vi "Execute_Analysis.vi"(0 "Image In":T2, 1 "ProjectName":string, 5 "Coordinate System Out (Set Coordinate System 1)":T3 {"Measurement System"."Axis Reference" items=["Direct", "Indirect"]; "Measurement System"."Angle (deg)" format="%.2f"; "Measurement System"."Origin"."Y" format="%.2f"; "Measurement System"."Origin"."X" format="%.2f"; "Reference System"."Axis Reference" items=["Direct", "Indirect"]; "Reference System"."Angle (deg)" format="%.2f"; "Reference System"."Origin"."Y" format="%.2f"; "Reference System"."Origin"."X" format="%.2f"}, 7 "ForCalCalculaton In":T2, 9 "ROI Entry":T4={"vROIName"="", "vROIContour"={"Contour Type"=0, "ROI Type"=0, "Points"=[]}, "ProcessSetting"=[], "Analysis_Setting"={"PreProcess"=enum."*Algorithm*", "Parameter"=""}}, 11 "error in (no error)":errorcluster, 12 "RootPath":path, 13 "CreatDllImage":bool, 14 "Script Index":i32) -> (4 "Image Out":T2, 6 "Result":variant, 8 "Analysis_Point_Result Out Overlay":T1[](array[typedef]), 10 "Analysis_Point_Result Out":T1[](array[typedef]), 15 "error out":errorcluster)   [LabVIEW 2019]
uses:
  Controls/Parttern Match/Analysis_PatternMatch_Parameter.ctl
  Controls/Barcode 1D/Analysis_Barcode 1D_Parameter.ctl
  <vilib>/vision/Instrument.llb/Demodulation Mode.ctl
  <vilib>/vision/Instrument.llb/Cell Sample Size.ctl
  <vilib>/vision/Instrument.llb/Cell Filter Mode.ctl
  <vilib>/vision/Instrument.llb/QR Code Search Options.ctl
  <vilib>/vision/Instrument.llb/Data Matrix Polarity.ctl
  <vilib>/vision/Instrument.llb/QR Code Model Type.ctl
  <vilib>/vision/Instrument.llb/QR Code Description Options.ctl
  Controls/Barcode 2D/Analysis_Barcode 2D_Parameter.ctl
  Controls/Clamp/Analysis_Clamp_Parameter.ctl
  Controls/Clamp MAX/Analysis_Clamp MAX_Parameter.ctl
  Controls/Particle/Analysis_Particle_Parameter.ctl
  Controls/Edge Detection/Analysis_Edge Detection_Parameter.ctl
  <vilib>/vision/NI_Vision_Development_Module.lvlib
  <vilib>/vision/Measure.llb/Edge Polarity.ctl
  <vilib>/vision/Measure.llb/Edge Options.ctl
  <vilib>/vision/Measure.llb/Straight Edge Process.ctl
  <vilib>/vision/Measure.llb/Straight Edge Options.ctl
  Controls/Find Straight Edge/Analysis_Find Straight Edge_Parameter.ctl
  <vilib>/vision/Instrument.llb/Data Matrix Search Options.ctl
  <vilib>/vision/Instrument.llb/Data Matrix Mirror.ctl
  <vilib>/vision/Instrument.llb/Cell Fill Percentage.ctl
  <vilib>/vision/Instrument.llb/ECC Type.ctl
  <vilib>/vision/Instrument.llb/Data Matrix Description Options.ctl
  DLL/[Global] Template.vi
  <vilib>/vision/Measure.llb/Edge New.ctl
  Controls/Parameter.ctl
  Controls/Histogram/Analysis_Histogram_Parameter.ctl
  Controls/Circle/Analysis_Circle_Parameter.ctl
  Controls/Parttern Match/Analysis_PatternMatch_ResultWithnumber.ctl
  Controls/ShapeDectect/Analysis_ShapeDectect_Parameter.ctl
  Controls/OCR/Analysis_OCR_Setting Parameter.ctl
  <vilib>/vision/Contour.llb/IMAQ Contour Curve Extraction.ctl
  <vilib>/vision/Contour.llb/IMAQ Connect Range Setting.ctl
  Controls/Contour/Analysis_Contour_Parameter.ctl
  Controls/ColorMatch/Analysis_ColorMatch_Parameter.ctl
  Controls/ColorMatch/Analysis_ColorMatch_Result.ctl
  <vilib>/vision/Instrument.llb/Data Matrix Advanced Options.ctl
  <vilib>/vision/Instrument.llb/Data Matrix Size Options.ctl
  Controls/Analysis_Type.ctl
  <vilib>/vision/Image Controls.llb/IMAQ Image.ctl
  Controls/Analysis_Setting.ctl
  Process/Controls/Process_Setting.ctl
  Controls/Vision_DataEntry.ctl
  Controls/Analysis_Result_To_Caliper.ctl
  Ctrl/VisionProcessName.ctl
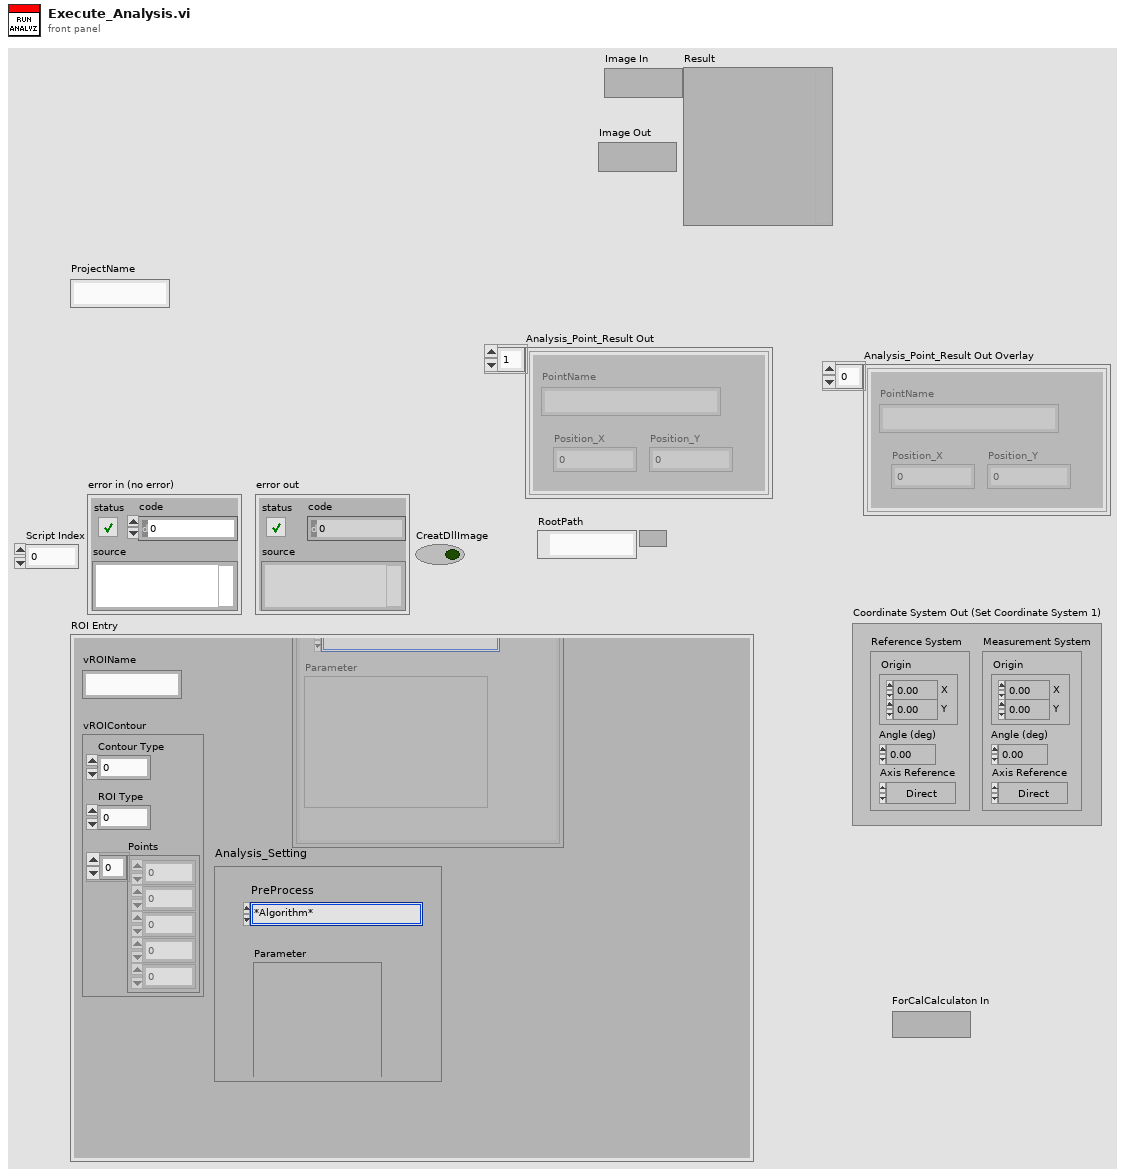
[diagram p1: front panel]
types:
  T1 = typedef "Analysis_Result_To_Caliper.ctl" = cluster{"PointName":string, "Position_X":dbl, "Position_Y":dbl}
  T2 = typedef "IMAQ Image.ctl" = refnum<image>
  T3 = cluster{"Reference System":cluster{"Origin":cluster{"X":sgl, "Y":sgl}, "Angle (deg)":sgl, "Axis Reference":u32}, "Measurement System":cluster{"Origin":cluster{"X":sgl, "Y":sgl}, "Angle (deg)":sgl, "Axis Reference":u32}}
  T4 = typedef "Vision_DataEntry.ctl" = cluster{"vROIName":string, "vROIContour":cluster{"Contour Type":u32, "ROI Type":u32, "Points":i32[]}, "ProcessSetting":T5[], "Analysis_Setting":T7}
  T5 = typedef "Process_Setting.ctl" = cluster{"Enum_PreProcess":T6, "Parameter":string}
  T6 = typedef "VisionProcessName.ctl" = enum16{"*CamParameter*", "CamAttributes", "*Preprocess*", "CG_Brightness", "C_Plane Extraction", "C_Threshold", "G_Lookup Table", "G_Threshold"}
  T7 = typedef "Analysis_Setting.ctl" = cluster{"PreProcess":T8, "Parameter":string}
  T8 = typedef "VisionProcessName.ctl" = enum16{"*CamParameter*", "CamAttributes", "*Preprocess*", "CG_Brightness", "C_Plane Extraction", "C_Threshold", "G_Lookup Table", "G_Threshold", "B_Image Inversion", "*Algorithm*", "CG_Histogram", "C_Color Matching", "C_Color Pattern Matching", "G_PatternMatch", "CG_Find Straight Edge", "CG_Adv. Find Straight Edge", "CG_Find Circular Edge", "G_Max Clamp", "G_Clamp (Rake)", "G_Pattern Matching"}
  T9 = typedef "Analysis_Type.ctl" = u16
  T10 = typedef "Parameter.ctl" = enum16{"Initialize", "Write", "Read", "WriteAll", "Save", "Load"}
  T11 = typedef "ParameterData.ctl" = cluster{"Rotate Angle":dbl, "Rotate?":bool, "Calibration File Path":string, "Cal?":bool}
  T12 = typedef "ROI Descriptor" = cluster{"Global Rectangle":i32[], "Contours":cluster{"ID":enum32{"External", "Internal"}, "Type":u32, "Coordinates":i32[]}[]}
  T13 = cluster{"Algorithm":i32, "Match Parameters":cluster{"Number of Matches Requested":i32, "Minimum Match Score":sgl, "Angle Ranges":cluster{"Start Angle":sgl, "End Angle":sgl}[]}, "ROI Descriptor":T12, "Advanced Options":cluster{"Item":u16, "Value":dbl}[], "Template path":string}
  T14 = typedef "Analysis_PatternMatch_ResultWithnumber.ctl" = cluster{"numbers":i32, "results":cluster{"ROI Descriptor out":T12, "Point":T15, "Angle":sgl, "Score":sgl, "Real World Coordinates":cluster{"X":sgl, "Y":sgl}, "Rectangle":T16}[]}
  T15 = typedef "IMAQ Point" = cluster{"X":sgl, "Y":sgl}
  T16 = typedef "IMAQ Rectangle" = cluster{"Left":i32, "Top":i32, "Right":i32, "Bottom":i32, "Rotation":dbl}
  T17 = typedef "Edge New.ctl" = cluster{"Location (Pixel)":cluster{"X":sgl, "Y":sgl}, "Location (Real-World)":cluster{"X":sgl, "Y":sgl}, "Distance (Pixel)":dbl, "Distance (Real-World)":dbl, "Strength":dbl, "Noise":dbl, "Rising?":bool}
  T18 = cluster{"Edge Information":T17[], "Number of Edges Detected":i32}
  T19 = cluster{cluster{"x":sgl, "y":sgl}[][], string[], "Barcodes":cluster{"Data":string, "Special Char 1":string, "Special Char 2":string, "Checksum(s)":string, "Barcode Type":u32, "Confidence Level":sgl, "Bounding Box":cluster{"x":sgl, "y":sgl}[]}[]}
  T20 = cluster{"Data":string, cluster{"x":sgl, "y":sgl}[]}
  T21 = cluster{"Points":cluster{"X":sgl, "Y":sgl}[], "Perpendicular Lines":cluster{cluster{sgl, sgl}, cluster{sgl, sgl}}[], "appended array":cluster{"X":sgl, "Y":sgl}[], "Line Coordinates":cluster{cluster{sgl, sgl}, cluster{sgl, sgl}}[], "Clamp Settings":cluster{"Contrast":i32, "Filter width":i32, "Steepness":i32, "Subsampling Ratio":u32, "Show Search Area":bool, "Show Search Lines":bool, "Show Edges Found":bool, "Show Result":bool}, "ROI Descriptor":cluster{"Global Rectangle":i32[], "Contours":cluster{"Contour Type":u32, "ROI Type":u32, "Points":i32[]}[]}, "Distance":sgl, "Edge Coordinates":cluster{"X":sgl, "Y":sgl}[], "Edge Coordinates  (Real World)":cluster{"X":sgl, "Y":sgl}[], "Distance (Real World)":sgl}
  T22 = cluster{cluster{"X":sgl, "Y":sgl}, cluster{"X":sgl, "Y":sgl}}
  T23 = cluster{"Area":dbl, "Number of Holes":dbl, "Bounding Rect":cluster{"Left":dbl, "Top":dbl, "Right":dbl, "Bottom":dbl}, "Center of Mass":cluster{"X":dbl, "Y":dbl}, "Orientation":dbl, "Dimensions":cluster{"Width":dbl, "Height":dbl}}
  T24 = cluster{"Left":dbl, "Top":dbl, "Right":dbl, "Bottom":dbl}
  T25 = cluster{"Point1 (Pixels)":cluster{"X":sgl, "Y":sgl}, "Point2 (Pixels)":cluster{"X":sgl, "Y":sgl}, "Point1 (Real-World)":cluster{"X":sgl, "Y":sgl}, "Point2 (Real-World)":cluster{"X":sgl, "Y":sgl}, "Angle (Pixel)":dbl, "Angle (Real-World)":dbl, "Score":dbl, "Straightness":dbl, "Average SNR (db)":dbl, "Calibration Valid":bool}
  T26 = typedef "IMAQ Circle" = cluster{"Center X":i32, "Center Y":i32, "Inner Radius":i32, "Outer Radius":i32, "Start Angle":dbl, "End Angle":dbl}
  T27 = typedef "Analysis_ShapeDectect_Parameter.ctl" = cluster{"Enum_ShapeType":enum16{"Circles", "Ellipses", "Lines", "Rectangles"}, "MaxParticle":i32, "Descriptor":cluster{"Set 1":dbl, "Set 2":dbl, "Set 3":dbl, "Set 4":dbl}, "Match Options":cluster{"Rotation":bool, "Scale":bool, "Occlusion":bool, "Range Settings":cluster{"Match Constraints":u32, "Min":dbl, "Max":dbl}[]}, "Curve Parameters":cluster{"Extraction Mode":u32, "Edge Threshold":i32, "Edge Filter Size":u32, "Min Length":i32, "Row Search Step Size":i32, "Col Search Step Size":i32, "Max Endpoint Gap":i32, "Closed":bool, "Subpixel":bool}, " score":dbl}
  T28 = typedef "Analysis_OCR_Setting Parameter.ctl" = cluster{"OCRSelectedLanaguage":string[]}
  T29 = typedef "Analysis_ColorMatch_Result.ctl" = cluster{"Match Flag":bool[], "Match Score":i32[], "ROI Descriptor":T12}
  T30 = typedef "Analysis_ColorMatch_Parameter.ctl" = cluster{"Color Sensitivity":u32, "Learn Saturation Threshold":i32, "Minimum Match Score":dbl, "Match Saturation Threshold":i32, "ROI Descriptor":T12, "TemplatePath":string, "ColorSpectrum":dbl[]}
  T31 = typedef "Analysis_PatternMatch_Parameter.ctl" = cluster{"Algorithm":i32, "Match Parameters":cluster{"Number of Matches Requested":i32, "Minimum Match Score":sgl, "Angle Ranges":cluster{"Start Angle":sgl, "End Angle":sgl}[]}, "ROI Descriptor":T12, "Advanced Options":cluster{"Item":u16, "Value":dbl}[], "Template path":string, "XOffset":i32, "YOffset":i32}
  T32 = typedef "Image Type" = u32
  T33 = cluster{"Number of Matches Requested":i32, "Minimum Match Score":sgl, "Angle Ranges":cluster{"Start Angle":sgl, "End Angle":sgl}[]}
  T34 = cluster{"Script Name":string, "TemplateArray":cluster{"ROI Name":string, "TemplateImage":T2}[]}[]
  T35 = cluster{"Script Name":string, "TemplateArray":cluster{"ROI Name":string, "TemplateImage":T2}[]}
  T36 = cluster{"Origin":cluster{"X":sgl, "Y":sgl}, "Angle (deg)":sgl, "Axis Reference":u32}
  T37 = typedef "Analysis_PatternMatch_Result.ctl" = cluster{"Position":cluster{"x":sgl, "y":sgl}, "Angle":sgl, "Scale":sgl, "Score":sgl, "Bounding Box":cluster{"x":sgl, "y":sgl}[]}
  T38 = cluster{"ROI Descriptor out":T12, "Point":T15, "Angle":sgl, "Score":sgl, "Real World Coordinates":cluster{"X":sgl, "Y":sgl}, "Rectangle":T16}
  T39 = typedef "Analysis_Edge Detection_Parameter.ctl" = cluster{"Edge Options":cluster{"Edge Polarity":u16, "Kernel Size":u32, "Width":u32, "Minimum Edge Strength":dbl, "Interpolation Type":u16, "Data Processing Method":u16}, "Process":u16, "Number of Matches Requested":i32, "ROI Descriptor":cluster{"Global Rectangle":i32[], "Contours":cluster{"Contour Type":u32, "ROI Type":u32, "Points":i32[]}[]}}
  T40 = cluster{"Edge Polarity":u16, "Kernel Size":u32, "Width":u32, "Minimum Edge Strength":dbl, "Interpolation Type":u16, "Data Processing Method":u16}
  T41 = cluster{"Global Rectangle":i32[], "Contours":cluster{"Contour Type":u32, "ROI Type":u32, "Points":i32[]}[]}
  T42 = cluster{"Contour Type":u32, "ROI Type":u32, "Points":i32[]}[]
  T43 = cluster{"Contour Type":u32, "ROI Type":u32, "Points":i32[]}
  T44 = typedef "Analysis_Barcode 1D_Parameter.ctl" = cluster{"Barcode Search Options":cluster{"Min Bar Width":dbl, "Min Edge Strength":dbl, "Min Bars":dbl, "Skip Location Search?":bool}, "Barcode Types To Search":enum16{"Reserved", "Codabar", "Code 39", "Code 93", "Code 128", "EAN 8", "EAN 13", "Interleaved 2 of 5", "MSI", "UPCA", "Pharmacode", "RSS Limited"}[], "Barcode Grading Options":cluster{"Calculate Grading Report":bool, "Scan Width ":dbl}, "Number of Matches Requested":i32, "ROI":cluster{"Global Rectangle":i32[], "Contours":cluster{"Contour Type":u32, "ROI Type":u32, "Points":i32[]}[]}}
  T45 = cluster{"Min Bar Width":dbl, "Min Edge Strength":dbl, "Min Bars":dbl, "Skip Location Search?":bool}
  T46 = enum16{"Reserved", "Codabar", "Code 39", "Code 93", "Code 128", "EAN 8", "EAN 13", "Interleaved 2 of 5", "MSI", "UPCA", "Pharmacode", "RSS Limited"}[]
  T47 = cluster{"Calculate Grading Report":bool, "Scan Width ":dbl}
  T48 = cluster{"Data":string, "Special Char 1":string, "Special Char 2":string, "Checksum(s)":string, "Barcode Type":u32, "Confidence Level":sgl, "Bounding Box":cluster{"x":sgl, "y":sgl}[]}[]
  T49 = cluster{T15[][], string[], "Barcodes":cluster{"Data":string, "Special Char 1":string, "Special Char 2":string, "Checksum(s)":string, "Barcode Type":u32, "Confidence Level":sgl, "Bounding Box":cluster{"x":sgl, "y":sgl}[]}[]}
  T50 = typedef "Analysis_Barcode 2D_Parameter.ctl" = cluster{"ROI":cluster{"Global Rectangle":i32[], "Contours":cluster{"Contour Type":u32, "ROI Type":u32, "Points":i32[]}[]}, "Barcode Type":enum16{"Data Matrix", "PDF417", "QR Code"}, "Data Matrix Parameter":cluster{"Data Matrix Description Options":T51, "Data Matrix Search Options":T56, "Data Matrix Size Options":T60, "Advanced Options":T61[]}, "PDF147 Search Mode":T62, "QR Code Parameter":cluster{"QR Search Options":T63, "QR Description Options":T64, "QR Code Cell Size (pixels)":cluster{"Minimum Size":u32, "Maximum Size":u32}}}
  T51 = typedef "Data Matrix Description Options.ctl" = cluster{"Aspect Ratio":sgl, "Rows":u32, "Columns":u32, "Rectangle":bool, "ECC":T52, "Barcode Polarity":T53, "Cell Fill Percentage":T54, "Minimum Border Integrity %":sgl, "Mirror Mode":T55}
  T52 = typedef "ECC Type.ctl" = i32
  T53 = typedef "Data Matrix Polarity.ctl" = i32
  T54 = typedef "Cell Fill Percentage.ctl" = i32
  T55 = typedef "Data Matrix Mirror.ctl" = i32
  T56 = typedef "Data Matrix Search Options.ctl" = cluster{"Rotation Mode":enum32{"Unlimited", "0 Degrees", "90 Degrees", "180 Degrees", "270 Degrees"}, "Skip Location?":bool, "Edge Threshold":u32, "Demodulation Mode":T57, "Cell Sample Size":T58, "Cell Filter Mode":T59, "Skew Degrees Allowed":u32, "Maximum Iterations":u32, "Initial Search Vector Width":u32}
  T57 = typedef "Demodulation Mode.ctl" = i32
  T58 = typedef "Cell Sample Size.ctl" = i32
  T59 = typedef "Cell Filter Mode.ctl" = i32
  T60 = typedef "Data Matrix Size Options.ctl" = cluster{"Data Matrix Size":cluster{"Minimum Size":u32, "Maximum Size":u32}, "Quiet Zone Width":u32}
  T61 = typedef "Data Matrix Advanced Options.ctl" = cluster{"Option":enum32{"Line Detection", "HighLight Filter", "Aggressive", "FNC1", "Refine Bounding Box"}, " Value":dbl}
  T62 = typedef "PDF417 Search Mode" = enum32{"Multiple Barcodes", "Single Barcode, Conservative"}
  T63 = typedef "QR Code Search Options.ctl" = cluster{"Rotation Mode":enum32{"Unlimited", "0 Degrees", "90 Degrees", "180 Degrees", "270 Degrees"}, "Skip Location?":bool, "Edge Threshold":u32, "Demodulation Mode":T57, "Cell Sample Size":T58, "Cell Filter Mode":T59, "Skew Degrees Allowed":u32}
  T64 = typedef "QR Code Description Options.ctl" = cluster{"Matrix Size (cells)":i32, "Barcode Polarity":T53, "Mirror Mode":i32, "QR Model":T65}
  T65 = typedef "QR Code Model Type.ctl" = i32
  T66 = cluster{"Data":string, "Bounding Box":cluster{"x":sgl, "y":sgl}[]}
  T67 = typedef "Analysis_Clamp_Parameter.ctl" = cluster{"Clamp Settings":cluster{"Contrast":i32, "Filter width":i32, "Steepness":i32, "Subsampling Ratio":u32, "Show Search Area":bool, "Show Search Lines":bool, "Show Edges Found":bool, "Show Result":bool}, "ROI Descriptor":cluster{"Global Rectangle":i32[], "Contours":cluster{"Contour Type":u32, "ROI Type":u32, "Points":i32[]}[]}, "Process":u16}
  T68 = cluster{"Contrast":i32, "Filter width":i32, "Steepness":i32, "Subsampling Ratio":u32, "Show Search Area":bool, "Show Search Lines":bool, "Show Edges Found":bool, "Show Result":bool}
  T69 = cluster{cluster{"X":sgl, "Y":sgl}, cluster{"X":sgl, "Y":sgl}}[]
  T70 = typedef "Analysis_Clamp MAX_Parameter.ctl" = cluster{"Overlay Settings":cluster{"Show Search Area":bool, "Show Curves":bool, "Show Clamp Locations":bool, "Show Result":bool, "Search Area Color":u32, "Curves Color":u32, "Clamp Locations Color":u32, "Result Color":u32, "Overlay Group Name":string}, "Curve Extraction Settings":cluster{"Extraction Mode":u32, "Edge Threshold":i32, "Edge Filter Size":u32, "Min Length":i32, "Row Search Step Size":i32, "Col Search Step Size":i32, "Max Endpoint Gap":i32, "Closed":bool, "Subpixel":bool}, "Clamp Settings":cluster{"Angle Range (+/-)":dbl, "Edge Polarity":cluster{"Start":u32, "End":u32}}, "ROI":cluster{"Global Rectangle":i32[], "Contours":cluster{"Contour Type":u32, "ROI Type":u32, "Points":i32[]}[]}}
  T71 = cluster{"Show Search Area":bool, "Show Curves":bool, "Show Clamp Locations":bool, "Show Result":bool, "Search Area Color":u32, "Curves Color":u32, "Clamp Locations Color":u32, "Result Color":u32, "Overlay Group Name":string}
  T72 = cluster{"Extraction Mode":u32, "Edge Threshold":i32, "Edge Filter Size":u32, "Min Length":i32, "Row Search Step Size":i32, "Col Search Step Size":i32, "Max Endpoint Gap":i32, "Closed":bool, "Subpixel":bool}
  T73 = cluster{"Angle Range (+/-)":dbl, "Edge Polarity":cluster{"Start":u32, "End":u32}}
  T74 = cluster{"Pixels ":cluster{"Start":cluster{"X":dbl, "Y":dbl}, "End":cluster{"X":dbl, "Y":dbl}}, "Real World":cluster{"Start":cluster{"X":dbl, "Y":dbl}, "End":cluster{"X":dbl, "Y":dbl}}}
  T75 = cluster{"Distance (Pixels)":dbl, "Distance (Real World)":dbl, "Angle (Absolute)":dbl, "Angle (Relative)":dbl}
  T76 = cluster{"Clamp Results":cluster{"Distance (Pixels)":dbl, "Distance (Real World)":dbl, "Angle (Absolute)":dbl, "Angle (Relative)":dbl}, "Clamp Points":cluster{"Pixels ":cluster{"Start":cluster{"X":dbl, "Y":dbl}, "End":cluster{"X":dbl, "Y":dbl}}, "Real World":cluster{"Start":cluster{"X":dbl, "Y":dbl}, "End":cluster{"X":dbl, "Y":dbl}}}}
  T77 = cluster{"Start":cluster{"X":dbl, "Y":dbl}, "End":cluster{"X":dbl, "Y":dbl}}
  T78 = typedef "Analysis_Particle_Parameter.ctl" = cluster{"Selected Particle":i32, "Connectivity 4/8 (8)":bool, "MaxParticle":i32}
  T79 = cluster{"Area":dbl, "Number of Holes":dbl, "Bounding Rect":cluster{"Left":dbl, "Top":dbl, "Right":dbl, "Bottom":dbl}, "Center of Mass":cluster{"X":dbl, "Y":dbl}, "Orientation":dbl, "Dimensions":cluster{"Width":dbl, "Height":dbl}}[]
  T80 = cluster{cluster{"Area":dbl, "Number of Holes":dbl, "Bounding Rect":cluster{"Left":dbl, "Top":dbl, "Right":dbl, "Bottom":dbl}, "Center of Mass":cluster{"X":dbl, "Y":dbl}, "Orientation":dbl, "Dimensions":cluster{"Width":dbl, "Height":dbl}}[], cluster{"Area":dbl, "Number of Holes":dbl, "Bounding Rect":cluster{"Left":dbl, "Top":dbl, "Right":dbl, "Bottom":dbl}, "Center of Mass":cluster{"X":dbl, "Y":dbl}, "Orientation":dbl, "Dimensions":cluster{"Width":dbl, "Height":dbl}}[]}
  T81 = typedef "Analysis_Histogram_Parameter.ctl" = cluster{"Interval Range":cluster{"Minimum":sgl, "Maximum":sgl}, "ROI Out":cluster{"Global Rectangle":i32[], "Contours":cluster{"Contour Type":u32, "ROI Type":u32, "Points":i32[]}[]}, "Number of Classes":i32}
  T82 = cluster{"histogram":u32[], "Minimal Value":sgl, "Maximal Value":sgl, "Starting Value":sgl, "Interval Width":sgl, "Mean Value":sgl, "Standard  Variation":sgl, "Area (pixels)":i32}
  T83 = cluster{"Histogram Report":cluster{"histogram":u32[], "Minimal Value":sgl, "Maximal Value":sgl, "Starting Value":sgl, "Interval Width":sgl, "Mean Value":sgl, "Standard  Variation":sgl, "Area (pixels)":i32}, "ROI Out":cluster{"Global Rectangle":i32[], "Contours":cluster{"Contour Type":u32, "ROI Type":u32, "Points":i32[]}[]}}
  T84 = typedef "Analysis_Find Straight Edge_Parameter.ctl" = cluster{"ROI Descriptor":cluster{"Global Rectangle":i32[], "Contours":cluster{"Contour Type":u32, "ROI Type":u32, "Points":i32[]}[]}, "Number of Matches Requested":i32, "Edge Info Size":i32, "Options":cluster{"Search Direction":u32, "Edge Options":T85, "Show Search Area":bool, "Show Search Lines":bool, "Show Edges Found":bool, "Show Result":bool, "Search Area Color":u32, "Search Lines Color":u32, "Edge Locations Color":u32, "Result Color":u32, "Overlay Group Name":string}, "Line Fit Options":T87}
  T85 = typedef "Edge Options.ctl" = cluster{"Edge Polarity":T86, "Kernel Size":u32, "Width":u32, "Minimum Edge Strength":sgl, "Interpolation Type":enum32{"Zero Order", "Bilinear", "Quadratic", "Cubic", "Bilinear Fixed"}, "Data Processing Method":enum32{"Average", "Median"}}
  T86 = typedef "Edge Polarity.ctl" = u32
  T87 = typedef "Straight Edge Options.ctl" = cluster{"Number of Lines":i32, "Type":T88, "Min. Score":dbl, "Max. Score":dbl, "Orientation":dbl, "Angle Range":dbl, "Angle Tolerance":dbl, "Step Size":u32, "Min. SNR (db)":dbl, "Min. Points (%)":dbl, "Hough Iterations":i32}
  T88 = typedef "Straight Edge Process.ctl" = enum32{"First Edge Rake", "Best Edge Rake", "Hough Edge Rake", "First Edge Projection", "Best Edge Projection"}
  T89 = cluster{"Search Direction":u32, "Edge Options":T85, "Show Search Area":bool, "Show Search Lines":bool, "Show Edges Found":bool, "Show Result":bool, "Search Area Color":u32, "Search Lines Color":u32, "Edge Locations Color":u32, "Result Color":u32, "Overlay Group Name":string}
  T90 = cluster{"Point1 (Pixels)":cluster{"X":sgl, "Y":sgl}, "Point2 (Pixels)":cluster{"X":sgl, "Y":sgl}, "Point1 (Real-World)":cluster{"X":sgl, "Y":sgl}, "Point2 (Real-World)":cluster{"X":sgl, "Y":sgl}, "Angle (Pixel)":dbl, "Angle (Real-World)":dbl, "Score":dbl, "Straightness":dbl, "Average SNR (db)":dbl, "Calibration Valid":bool}[]
  T91 = typedef "Analysis_Circle_Parameter.ctl" = cluster{"ROI Descriptor":cluster{"Global Rectangle":i32[], "Contours":cluster{"Contour Type":u32, "ROI Type":u32, "Points":i32[]}[]}, "Options":cluster{"Search  Direction":u32, "Edge Options":T85, "Show Search Area":bool, "Show Search Lines":bool, "Show Edges Found":bool, "Show Result":bool, "Search Area Color":u32, "Search Lines Color":u32, "Edge Locations Color":u32, "Result Color":u32, "Overlay Group Name":string}, "Circle Fit Options":cluster{"Process":enum16{"Get First Edge", "Get First + Last Edge", "Get All Edges", "Get Best Edge"}, "Step Size":dbl, "Max Pixel Radius":i32}}
  T92 = cluster{"Search  Direction":u32, "Edge Options":T85, "Show Search Area":bool, "Show Search Lines":bool, "Show Edges Found":bool, "Show Result":bool, "Search Area Color":u32, "Search Lines Color":u32, "Edge Locations Color":u32, "Result Color":u32, "Overlay Group Name":string}
  T93 = cluster{"Process":enum16{"Get First Edge", "Get First + Last Edge", "Get All Edges", "Get Best Edge"}, "Step Size":dbl, "Max Pixel Radius":i32}
  T94 = cluster{"Center (Pixels)":cluster{"X":sgl, "Y":sgl}, "Radius (Pixels)":dbl, "Center (Real-World)":cluster{"X":sgl, "Y":sgl}, "Radius (Real-World)":dbl, "Roundness (Real-World)":dbl, "Average Strength":dbl, "Average SNR (dB)":dbl}
  T95 = cluster{"ROI Descriptor out":T12, "ROI Descriptor out":T12, "Fitted Circle":cluster{"Center (Pixels)":cluster{"X":sgl, "Y":sgl}, "Radius (Pixels)":dbl, "Center (Real-World)":cluster{"X":sgl, "Y":sgl}, "Radius (Real-World)":dbl, "Roundness (Real-World)":dbl, "Average Strength":dbl, "Average SNR (dB)":dbl}}
  T96 = cluster{"Pixel":cluster{"Position":cluster{"X":sgl, "Y":sgl}, "Angle":dbl, "Major Radius":dbl, "Minor Radius":dbl, "Score":dbl}[], "Ellipses (Calibrated)":cluster{"Position":cluster{"X":sgl, "Y":sgl}, "Orientation":dbl, "Major Radius":dbl, "Minor Radius":dbl, "Score":dbl}[]}
  T97 = enum16{"Circles", "Ellipses", "Lines", "Rectangles"}
  T98 = cluster{"Circles":cluster{"Position":cluster{"X":sgl, "Y":sgl}, "Radius":dbl, "Score":dbl}[], "Circles (Calibrated)":cluster{"Position":cluster{"X":sgl, "Y":sgl}, "Radius":dbl, "Score":dbl}[]}
  T99 = cluster{"Position":cluster{"X":sgl, "Y":sgl}, "Radius":dbl, "Score":dbl}[]
  T100 = cluster{"Position":cluster{"X":sgl, "Y":sgl}, "Radius":dbl, "Score":dbl}
  T101 = cluster{"ROI Descriptor out":T12, "Circle Descriptor":cluster{"Position":cluster{"X":sgl, "Y":sgl}, "Radius":dbl, "Score":dbl}, "Circle Descriptor":cluster{"Position":cluster{"X":sgl, "Y":sgl}, "Radius":dbl, "Score":dbl}}
  T102 = cluster{"Enum_ShapeType":enum16{"Circles", "Ellipses", "Lines", "Rectangles"}, "DectectItem":i32, cluster{"ROI Descriptor out":T12, "Circle Descriptor":cluster{"Position":cluster{"X":sgl, "Y":sgl}, "Radius":dbl, "Score":dbl}, "Circle Descriptor":cluster{"Position":cluster{"X":sgl, "Y":sgl}, "Radius":dbl, "Score":dbl}}[]}
  T103 = cluster{"Position":cluster{"X":sgl, "Y":sgl}, "Angle":dbl, "Major Radius":dbl, "Minor Radius":dbl, "Score":dbl}[]
  T104 = cluster{"Position":cluster{"X":sgl, "Y":sgl}, "Orientation":dbl, "Major Radius":dbl, "Minor Radius":dbl, "Score":dbl}[]
  T105 = cluster{"Position":cluster{"X":sgl, "Y":sgl}, "Angle":dbl, "Major Radius":dbl, "Minor Radius":dbl, "Score":dbl}
  T106 = cluster{"Position":cluster{"X":sgl, "Y":sgl}, "Orientation":dbl, "Major Radius":dbl, "Minor Radius":dbl, "Score":dbl}
  T107 = cluster{"ROI Descriptor out":T12, "Circle Descriptor":cluster{"Position":cluster{"X":sgl, "Y":sgl}, "Angle":dbl, "Major Radius":dbl, "Minor Radius":dbl, "Score":dbl}, "Circle Descriptor":cluster{"Position":cluster{"X":sgl, "Y":sgl}, "Orientation":dbl, "Major Radius":dbl, "Minor Radius":dbl, "Score":dbl}}
  T108 = cluster{"Enum_ShapeType":enum16{"Circles", "Ellipses", "Lines", "Rectangles"}, "DectectItem":i32, cluster{"ROI Descriptor out":T12, "Circle Descriptor":cluster{"Position":cluster{"X":sgl, "Y":sgl}, "Angle":dbl, "Major Radius":dbl, "Minor Radius":dbl, "Score":dbl}, "Circle Descriptor":cluster{"Position":cluster{"X":sgl, "Y":sgl}, "Orientation":dbl, "Major Radius":dbl, "Minor Radius":dbl, "Score":dbl}}[]}
  T109 = cluster{"Lines":cluster{"Start Point":cluster{"X":sgl, "Y":sgl}, "End Point":cluster{"X":sgl, "Y":sgl}, "Length":dbl, "Angle":dbl, "Score":dbl}[], "Lines Calibrated":cluster{"Start Point":cluster{"X":sgl, "Y":sgl}, "End Point":cluster{"X":sgl, "Y":sgl}, "Length":dbl, "Orientation":dbl, "Score":dbl}[]}
  T110 = cluster{"Start Point":cluster{"X":sgl, "Y":sgl}, "End Point":cluster{"X":sgl, "Y":sgl}, "Length":dbl, "Angle":dbl, "Score":dbl}[]
  T111 = cluster{"Start Point":cluster{"X":sgl, "Y":sgl}, "End Point":cluster{"X":sgl, "Y":sgl}, "Length":dbl, "Orientation":dbl, "Score":dbl}[]
  T112 = cluster{"Start Point":cluster{"X":sgl, "Y":sgl}, "End Point":cluster{"X":sgl, "Y":sgl}, "Length":dbl, "Angle":dbl, "Score":dbl}
  T113 = cluster{"Start Point":cluster{"X":sgl, "Y":sgl}, "End Point":cluster{"X":sgl, "Y":sgl}, "Length":dbl, "Orientation":dbl, "Score":dbl}
  T114 = cluster{"Circle Descriptor":cluster{"Start Point":cluster{"X":sgl, "Y":sgl}, "End Point":cluster{"X":sgl, "Y":sgl}, "Length":dbl, "Angle":dbl, "Score":dbl}, "Circle Descriptor":cluster{"Start Point":cluster{"X":sgl, "Y":sgl}, "End Point":cluster{"X":sgl, "Y":sgl}, "Length":dbl, "Orientation":dbl, "Score":dbl}}
  T115 = cluster{"Enum_ShapeType":enum16{"Circles", "Ellipses", "Lines", "Rectangles"}, "DectectItem":i32, cluster{"Circle Descriptor":cluster{"Start Point":cluster{"X":sgl, "Y":sgl}, "End Point":cluster{"X":sgl, "Y":sgl}, "Length":dbl, "Angle":dbl, "Score":dbl}, "Circle Descriptor":cluster{"Start Point":cluster{"X":sgl, "Y":sgl}, "End Point":cluster{"X":sgl, "Y":sgl}, "Length":dbl, "Orientation":dbl, "Score":dbl}}[]}
  T116 = cluster{"Rectangles":cluster{"Corners":cluster{"X":sgl, "Y":sgl}[], "Angle":dbl, "Width":dbl, "Height":dbl, "Score":dbl}[], "Rectangles Calibrated":cluster{"Corners":cluster{"X":sgl, "Y":sgl}[], "Angle":dbl, "Width":dbl, "Height":dbl, "Score":dbl}[]}
  T117 = cluster{"Corners":cluster{"X":sgl, "Y":sgl}[], "Angle":dbl, "Width":dbl, "Height":dbl, "Score":dbl}[]
  T118 = cluster{"Corners":cluster{"X":sgl, "Y":sgl}[], "Angle":dbl, "Width":dbl, "Height":dbl, "Score":dbl}
  T119 = cluster{"Rectangle Descriptor":cluster{"Corners":cluster{"X":sgl, "Y":sgl}[], "Angle":dbl, "Width":dbl, "Height":dbl, "Score":dbl}, "Rectangle Descriptor":cluster{"Corners":cluster{"X":sgl, "Y":sgl}[], "Angle":dbl, "Width":dbl, "Height":dbl, "Score":dbl}}
  T120 = cluster{"Enum_ShapeType":enum16{"Circles", "Ellipses", "Lines", "Rectangles"}, "DectectItem":i32, cluster{"Rectangle Descriptor":cluster{"Corners":cluster{"X":sgl, "Y":sgl}[], "Angle":dbl, "Width":dbl, "Height":dbl, "Score":dbl}, "Rectangle Descriptor":cluster{"Corners":cluster{"X":sgl, "Y":sgl}[], "Angle":dbl, "Width":dbl, "Height":dbl, "Score":dbl}}[]}
  T121 = typedef "Analysis_Contour_Parameter.ctl" = cluster{"ROI":cluster{"Global Rectangle":i32[], "Contours":cluster{"ID":enum32{"External", "Internal"}, "Type":u32, "Coordinates":i32[]}[]}, "Search Direction":enum16{"Rect Left To Right", "Rect Right To Left", "Rect Top To Bottom", "Rect Bottom To Top", "Annulus Inner To Outer", "Annulus Outer To Inner", "Annulus Start Angle To End Angle", "Annulus End Angle To Start Angle"}, "Curve Extraction":T122, "Contour Selection":enum16{"Closest To Search Start", "Maximum Length", "Strongest Mean Gradient Change"}, "Curve Connection":T123[]}
  T122 = typedef "IMAQ Contour Curve Extraction.ctl" = cluster{"Extraction Mode":u32, "Edge Threshold":i32, "Edge Filter Size":u32, "Min Length":i32, "Search Step Size":i32, "Max Endpoint Gap":i32, "Subpixel":bool}
  T123 = typedef "IMAQ Connect Range Setting.ctl" = cluster{"Match Constraints":u32, "Min":dbl, "Max":dbl}
  T124 = typedef "Analysis_Contour_Result.ctl" = cluster{"Points (pixel)":cluster{"X":dbl, "Y":dbl}[], "Points (real)":cluster{"X":dbl, "Y":dbl}[], "Length (pixel)":dbl, "Length (real)":dbl}
  T125 = cluster{"ID":enum32{"External", "Internal"}, "Type":u32, "Coordinates":i32[]}[]
  T126 = cluster{"ID":enum32{"External", "Internal"}, "Type":u32, "Coordinates":i32[]}
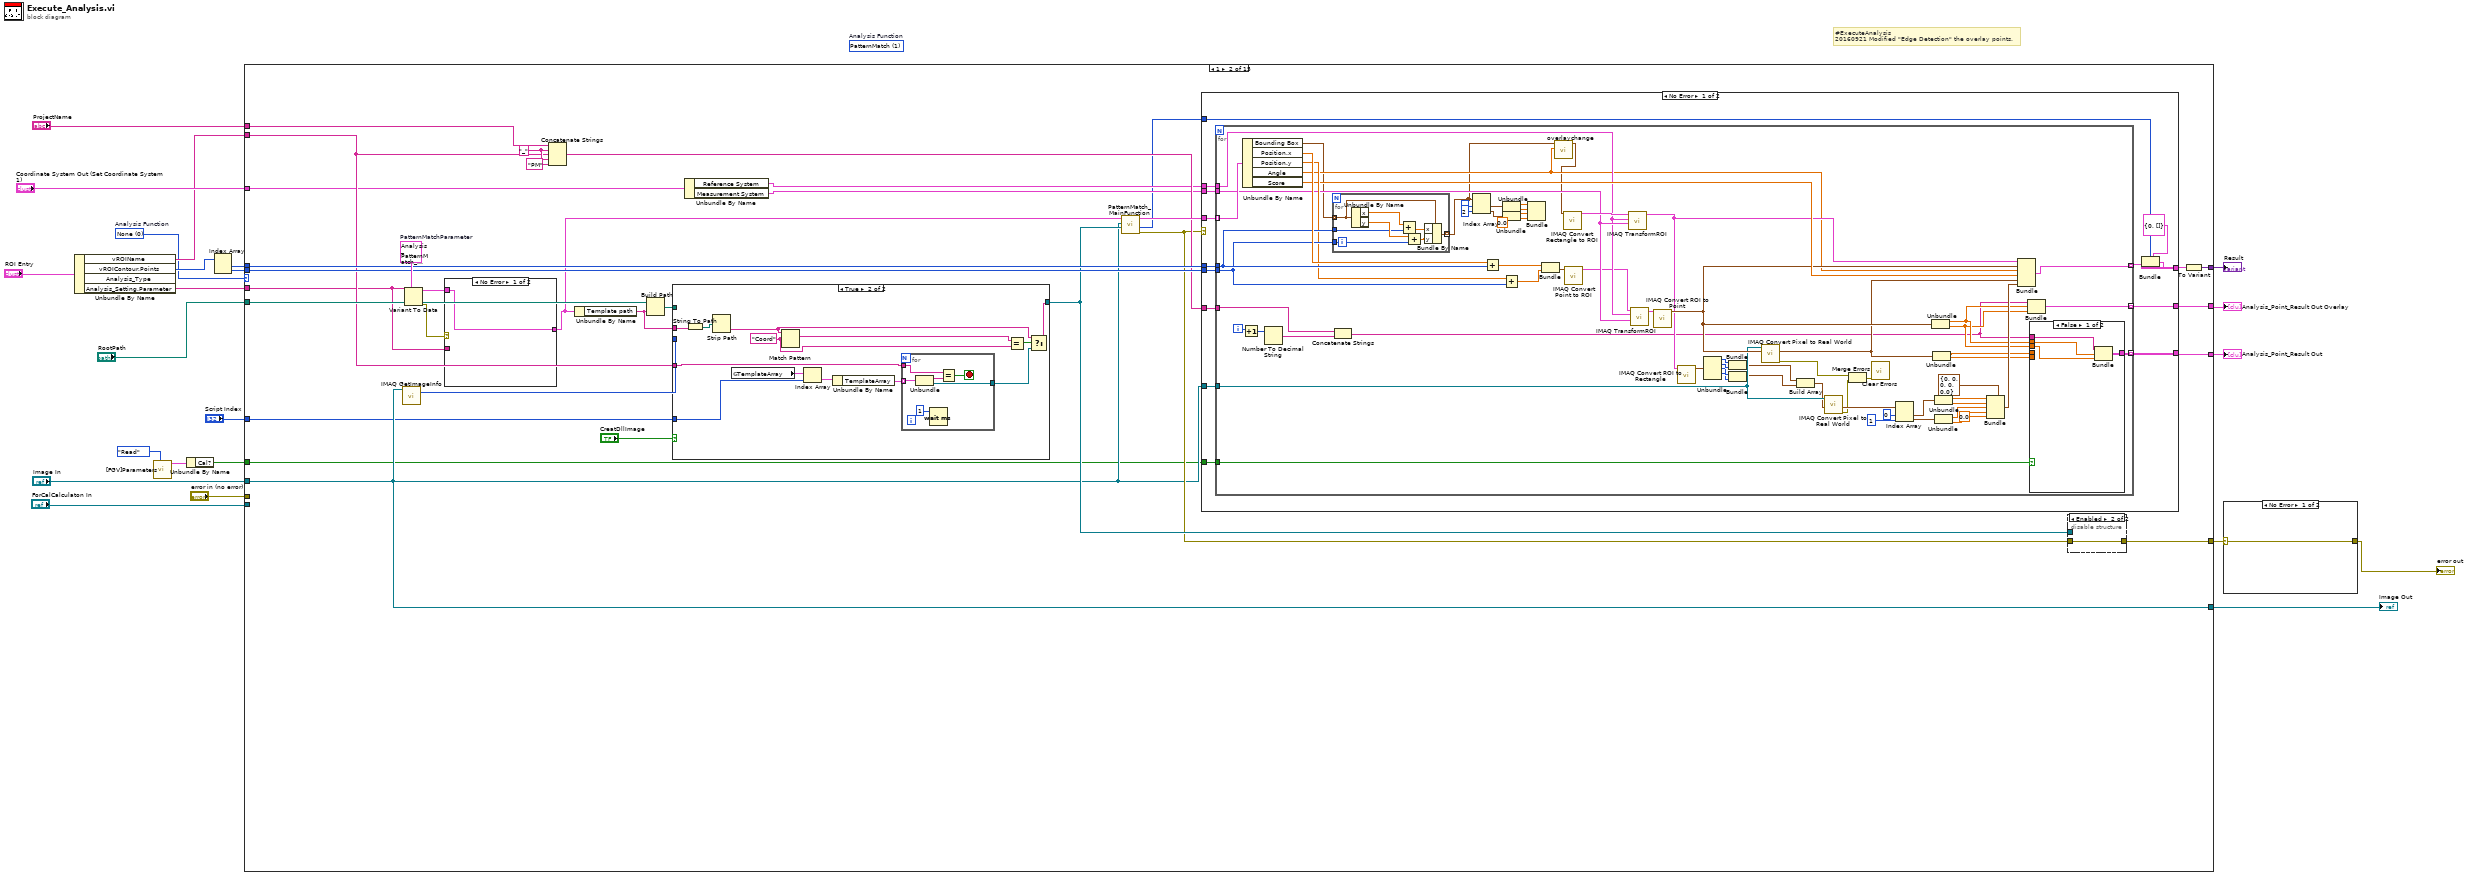
[diagram p0: block diagram]
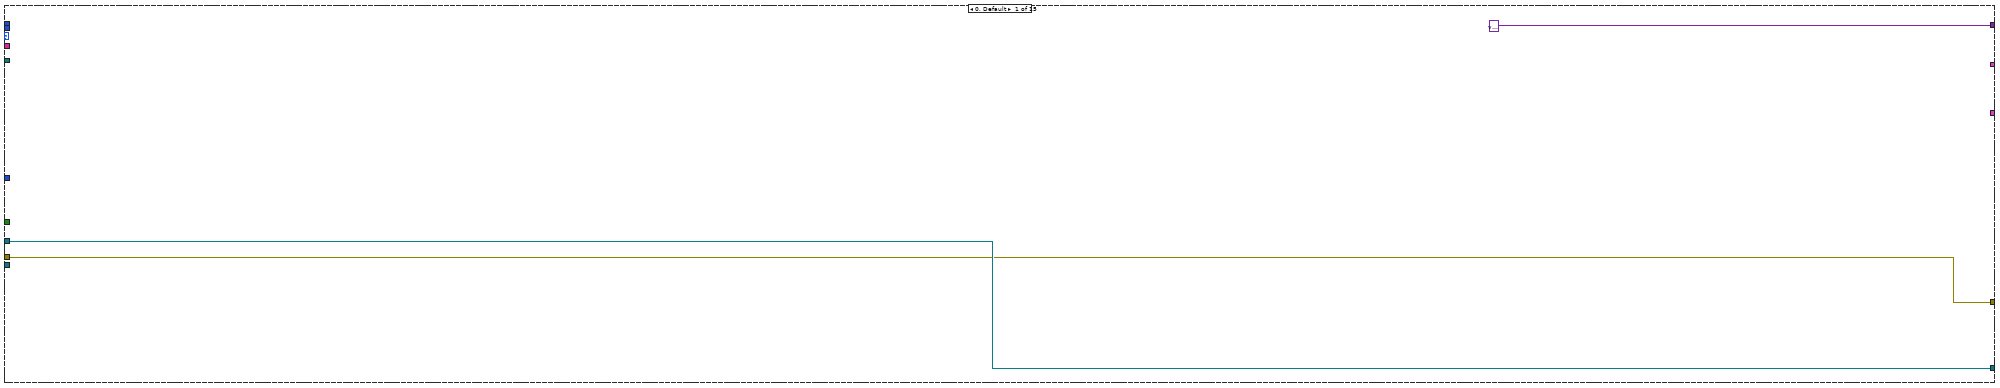
[diagram p3: hidden frame]
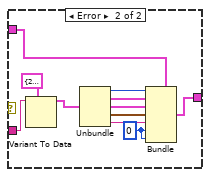
[diagram p4: hidden frame]
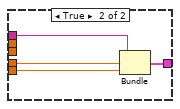
[diagram p5: hidden frame]
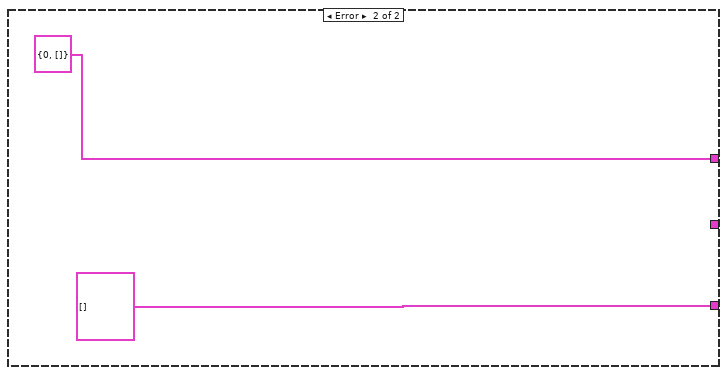
[diagram p6: hidden frame]
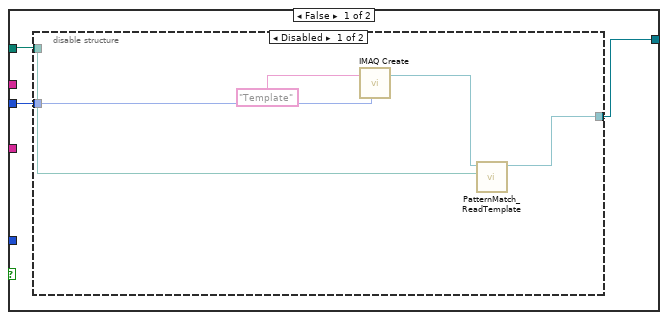
[diagram p7: hidden frame]
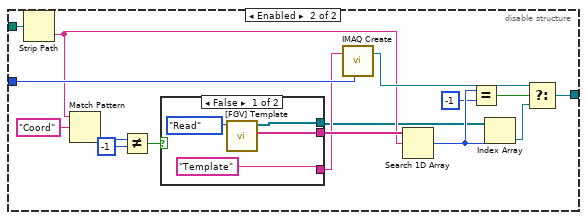
[diagram p8: hidden frame]
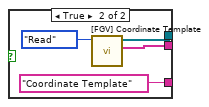
[diagram p9: hidden frame]
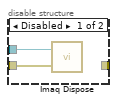
[diagram p10: hidden frame]
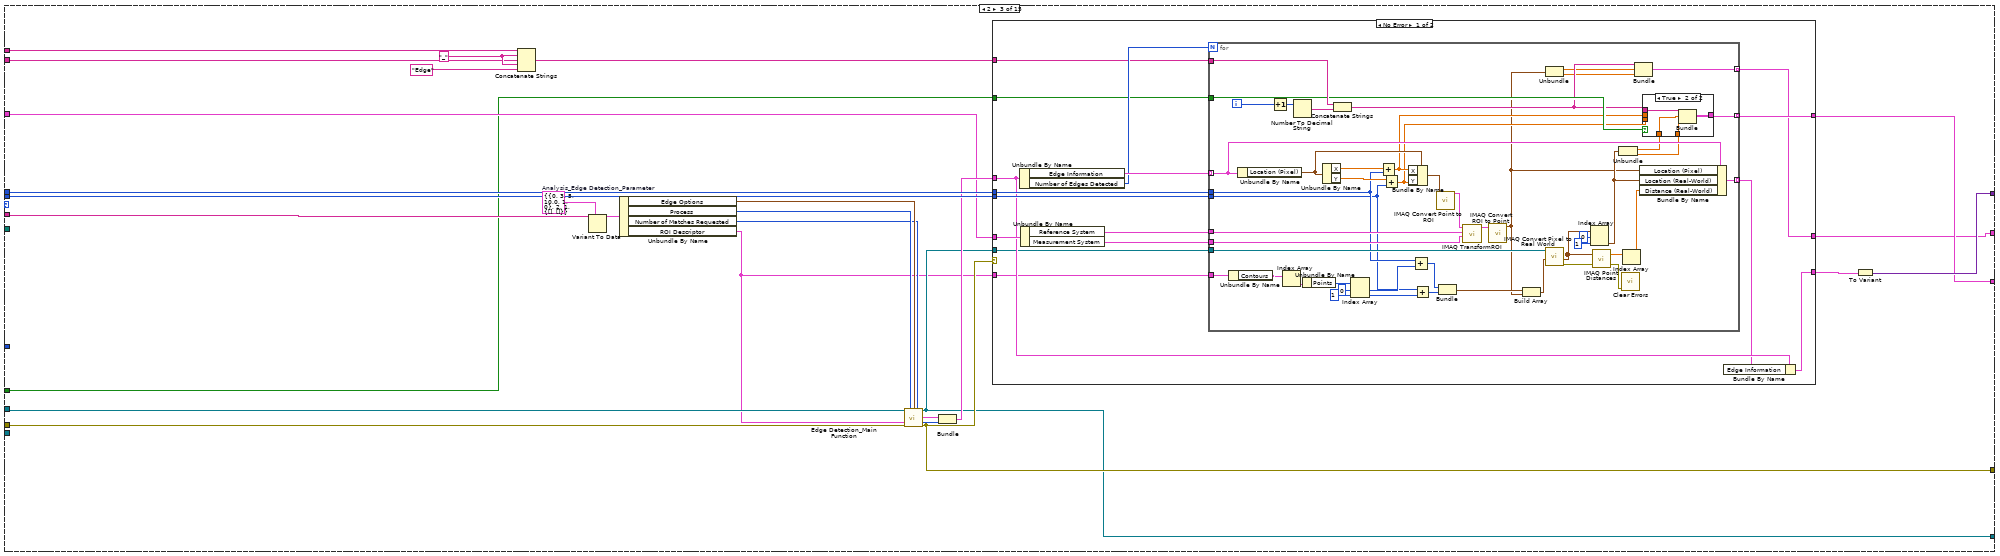
[diagram p11: hidden frame]
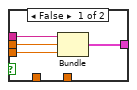
[diagram p12: hidden frame]
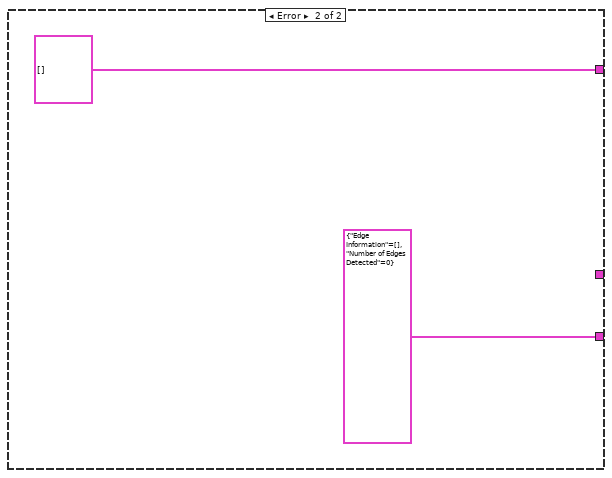
[diagram p13: hidden frame]
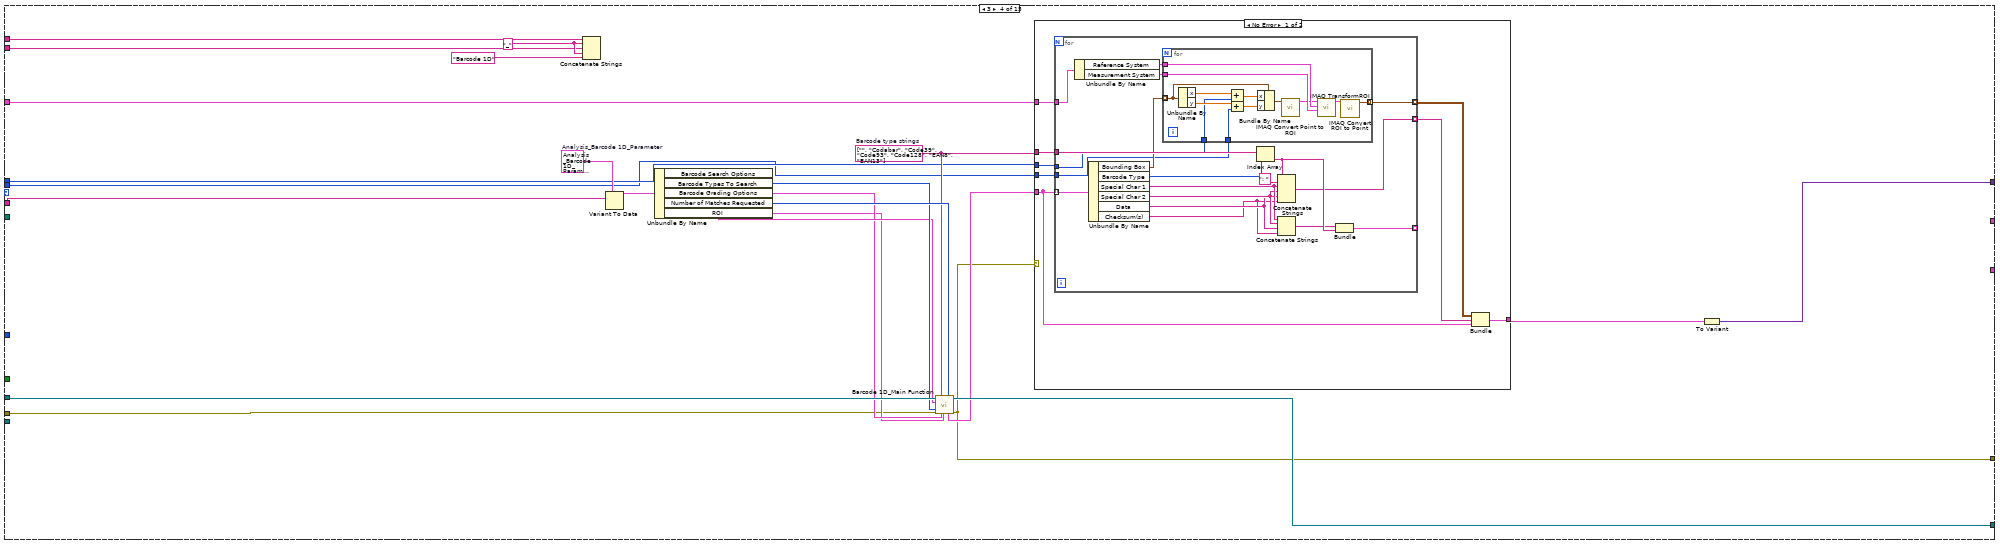
[diagram p14: hidden frame]
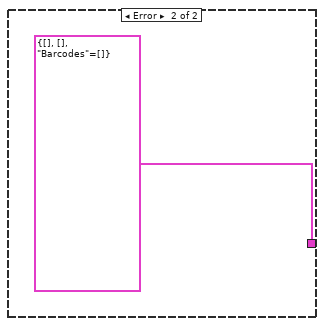
[diagram p15: hidden frame]
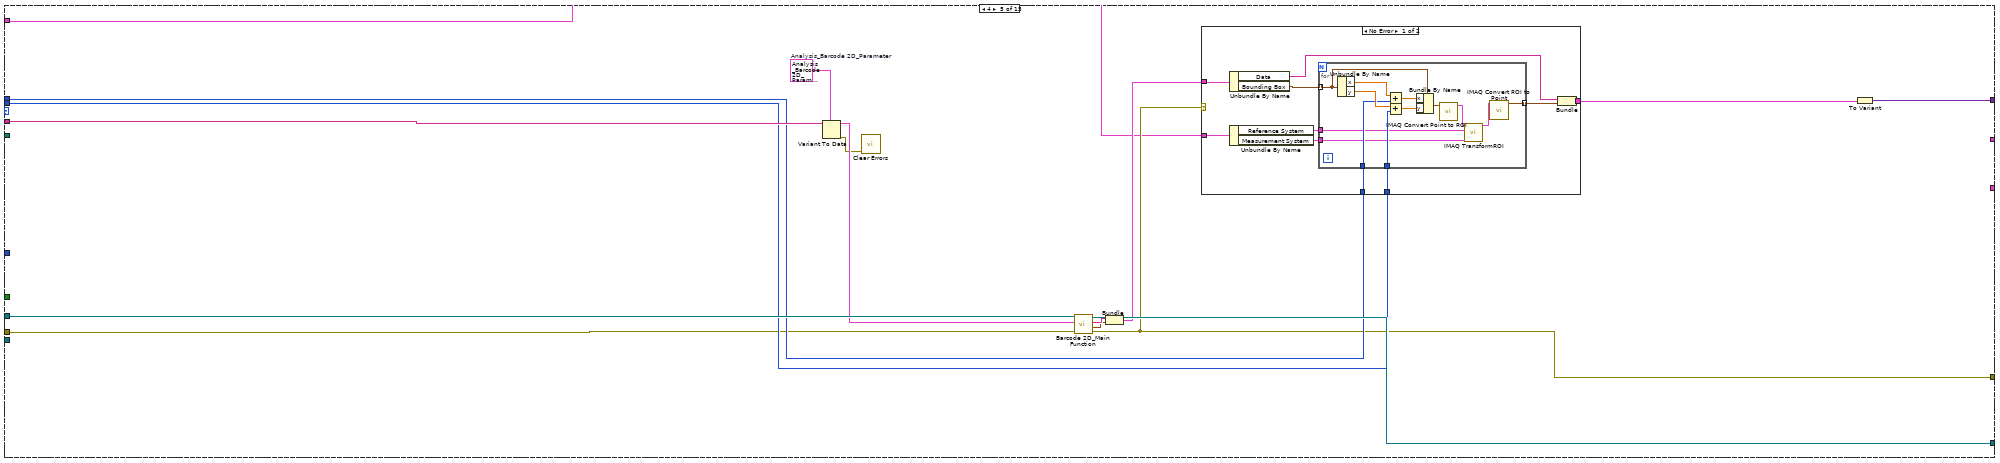
[diagram p16: hidden frame]
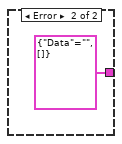
[diagram p17: hidden frame]
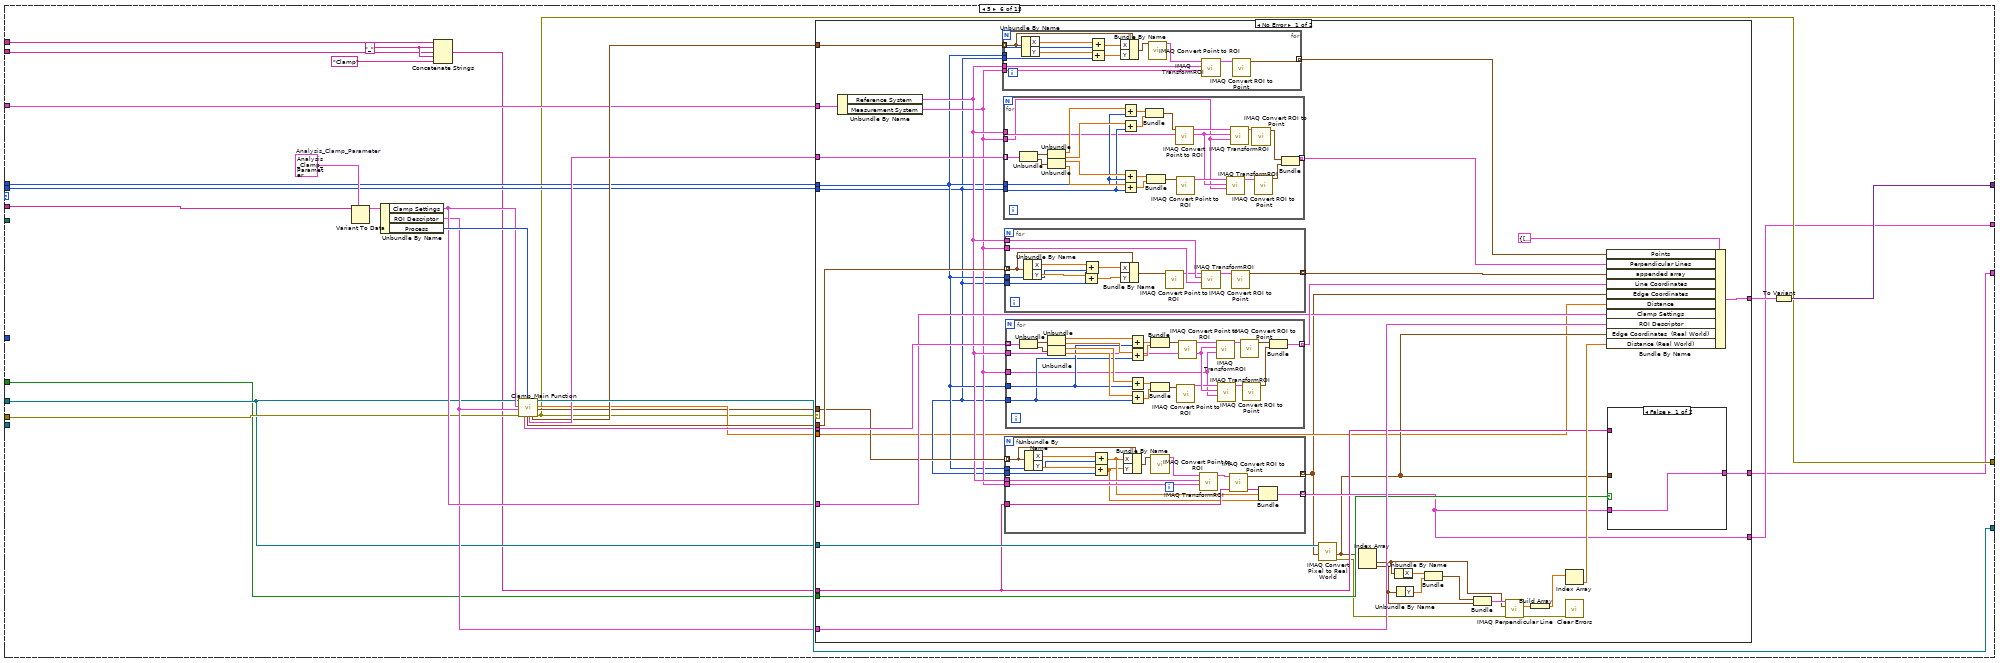
[diagram p18: hidden frame]
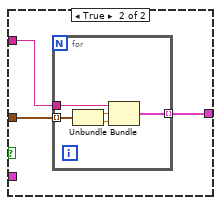
[diagram p19: hidden frame]
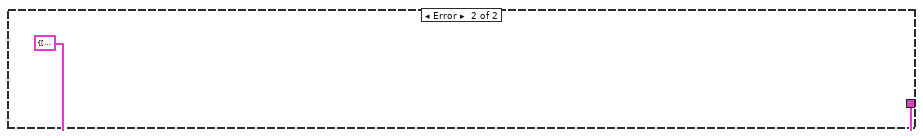
[diagram p20: hidden frame]
diagram:
  (unwired) T9 1 items=["None", "PatternMatch", "Edge Detection", "Barcode 1D", "Barcode 2D", "Clamp", "Clamp MAX", "Particle", "Histogram", "Straight Edge", "Circle", "Shape Detect", "OCR", "Contour", "ColorMatch"]  # Analysis Function
  w1 = T9 0 items=["None", "PatternMatch", "Edge Detection", "Barcode 1D", "Barcode 2D", "Clamp", "Clamp MAX", "Particle", "Histogram", "Straight Edge", "Circle", "Shape Detect", "OCR", "Contour", "ColorMatch"]  # Analysis Function
  # "#ExecuteAnalysis\n20160921 Modified \"Edge Detection\" the overlay points."
  n1 = Unbundle By Name("ROI Entry") -> ("vROIName"=w11:string, "vROIContour.Points"=w18:i32[], "Analysis_Setting.Parameter"=w12:string)  [unwired: 1 out]
  n2 = call "[FGV]Parameters.vi"("Parameter"=Parameter."Read") -> ("ParameterData Out"=w5:T11)  [unwired: 9 in, 1 out]
  n3 = Unbundle By Name(w5) -> ("Cal?"=w4:bool)
  n4 = Index Array(array=w18) -> (element #1=w21:i32, element #2=w20:i32)  [unwired: 2 in]
  n5 = case shown="1" w1 {
    tunnel: w12 -> [_ w27 w248 w346 w403 w456 w622 w721 w808 w830 w981 w983 w1284 w1344 w1392]
    tunnel: "Image In" -> [w26 w43 w249 w342 w401 w437 w621 w718 w804 w817 w978 w984 w1286 w1342 w1391]
    tunnel: [w26 w43 w226 w337 w397 w451 w606 w710 w801 w813 w937 _ w1286 w1328 w1379] -> w23
    tunnel: [variant ("Variant") w54 w242 w333 w398 w453 w610 w714 w807 w820 w973 w988 w1285 w1327 w1382] -> w22
    tunnel: w21 -> [_ w56 w239 w332 w394 w446 w612 w716 _ w824 w964 w995 _ w1341 w1373]
    tunnel: w20 -> [_ w55 w238 w331 w393 w445 w611 w715 _ w823 w963 w994 _ w1340 w1370]
    tunnel: "Coordinate System Out (Set Coordinate System 1)" -> [_ w35 w227 w324 w390 w438 w607 w711 _ w814 w972 w1003 _ w1336 w1390]
    tunnel: w11 -> [_ w36 w233 w328 _ w432 w597 w701 _ w809 w950 w999 w1291 _ _]
    tunnel: [_ w52 w231 _ _ w428 w595 w698 _ w821 w939 w990 _ _ _] -> w16
    tunnel: "ProjectName" -> [_ w42 w230 w327 _ w433 w598 w700 _ w831 w951 w1000 w1293 _ _]
    tunnel: "RootPath" -> [_ w51 _ _ _ _ _ _ _ _ _ _ _ _ _]
    tunnel: "error in (no error)" -> [w24 _ w229 w326 w392 w439 w609 w713 w798 w816 w975 w986 _ _ _]
    tunnel: [w24 w45 w228 w325 w391 w436 w608 w712 w797 w815 _ _ _ _ _] -> w9
    tunnel: "ForCalCalculaton In" -> [_ _ _ _ _ _ _ w706 _ _ _ _ _ _ w1380]
    tunnel: w4 -> [_ w41 w224 _ _ w430 w594 w704 _ w812 _ w985 _ w1333 w1381]
    tunnel: [_ w40 w223 _ _ w429 w593 w697 _ w811 w941 w992 _ _ _] -> w3
    tunnel: "Script Index" -> [_ w39 _ _ _ _ _ _ _ _ _ _ _ _ _]
    frame 0, Default {
    }
    frame 1 {
      w38 = "_" ("string")
      w58 = T31 {"Algorithm"=2, "Match Parameters"={"Number of Matches Requested"=1, "Minimum Match Score"=750.0, "Angle Ranges"=[]}, "ROI Descriptor"={"Global Rectangle"=[], "Contours"=[]}, "Advanced Options"=[{"Item"=1, "Value"=1.0}, {"Item"=103, "Value"=1.0}], "Template path"="", "XOffset"=0, "YOffset"=0}  # PatternMatchParameter
      n6 = call "IMAQ GetImageInfo"("Image"=w43) -> ("Image Type"=w49:T32)  [unwired: 3 in, 7 out]
      n7 = Variant To Data(type=w58, Variant=w27) -> (data=w29:T31, error out=w30:errorcluster)  [unwired: 1 in]
      n8 = case shown="No Error" w30 {
        tunnel: w27 -> [_ w69]
        tunnel: [w59 w67] -> w28
        tunnel: w29 -> [w59 w68]
        frame No Error {
        }
        frame Error {
          w60 = 0 ("XOffset")
          n9 = Variant To Data(type=T13 {"Algorithm"=2, "Match Parameters"={"Number of Matches Requested"=1, "Minimum Match Score"=750.0, "Angle Ranges"=[]}, "ROI Descriptor"={"Global Rectangle"=[], "Contours"=[]}, "Advanced Options"=[{"Item"=1, "Value"=1.0}, {"Item"=103, "Value"=1.0}], "Template path"=""} ("PatternMatchParameter"), Variant=w69) -> (data=w66:T13)  [unwired: 1 in, 1 out]
          n10 = Unbundle(w66) -> ("Algorithm"=w65:i32, "Match Parameters"=w64:T33, "ROI Descriptor"=w63:T12, "Advanced Options"=w62:cluster{"Item":u16, "Value":dbl}[], "Template path"=w61:string)
          n11 = Bundle(cluster=w68, "Algorithm"=w65, "Match Parameters"=w64, "ROI Descriptor"=w63, "Advanced Options"=w62, "Template path"=w61, "XOffset"=w60, "YOffset"=w60) -> (w67:T31)
        }
      }
      n12 = Concatenate Strings(w42, w38, w36, w38, "PM" ("string")) -> (w46:string)
      n13 = Unbundle By Name(w28) -> ("Template path"=w31:string)
      n14 = Build Path(base path=w51, name or relative path=w31) -> (appended path=w48:path)
      n15 = case shown="True" "CreatDllImage" {
        tunnel: w49 -> [w171 _]
        tunnel: w48 -> [w170 _]
        tunnel: [w169 w201] -> w47
        tunnel: w36 -> [_ w207]
        tunnel: w39 -> [_ w210]
        tunnel: w31 -> [_ w209]
        frame False {
          n16 = disable-structure shown="Disabled" {
            disable-tunnel: w171 -> [w175 w192]
            disable-tunnel: w170 -> [w174 w190]
            disable-tunnel: [w172 w191] -> w169
            frame Disabled {
              n17 = call "IMAQ Create"("Image Name"="Template", "Image Type"=w175) -> ("New Image"=w173:T2)  [unwired: 2 in, 2 out]
              n18 = call "PatternMatch_ReadTemplate.vi"("template path"=w174, "Template"=w173) -> ("Template Out"=w172:T2)  [unwired: 8 in, 1 out]
            }
            frame Enabled {
              n19 = Strip Path(path=w190) -> (name=w183:string)  [unwired: 1 out]
              n20 = Match Pattern(string=w183, regular expression="Coord") -> (offset past match=w181:i32)  [unwired: 1 in, 3 out]
              n21 = Not Equal?(x=w181, y=-1) -> (x != y?=w179:bool)
              n22 = case shown="False" w179 {
                tunnel: [w196 w199] -> w177
                tunnel: [w195 w198] -> w184
                tunnel: ["Template" ("Image Name") "Coordinate Template"] -> w178
                frame False {
                  n23 = call "[FGV] Template.vi"("Command"=enum16{"Initialize", "Save", "Read"}."Read") -> ("Image Name Array"=w195:string[], "Image Array"=w196:T2[])  [unwired: 8 in, 1 out]
                }
                frame True {
                  n24 = call "[FGV] Coordinate Template.vi"("Command"=enum16{"Initialize", "Save", "Read"}."Read") -> ("Image Name Array"=w198:string[], "Image Array"=w199:T2[])  [unwired: 8 in, 1 out]
                }
              }
              n25 = call "IMAQ Create"("Image Name"=w178, "Image Type"=w192) -> ("New Image"=w185:T2)  [unwired: 2 in, 2 out]
              n26 = Search 1D Array(1D array=w184, element=w183) -> (index of element=w189:i32)  [unwired: 1 in]
              n27 = Equal?(x=w189, y=-1) -> (x = y?=w187:bool)
              n28 = Index Array(array=w177, index=w189) -> (element=w186:T2)
              n29 = Select(t=w185, s=w187, f=w186) -> (s? t:f=w191:T2)
            }
          }
        }
        frame True {
          w205 = "Coord" ("regular expression")
          n30 = String To Path(string=w209) -> (path=w208:path)
          n31 = Strip Path(path=w208) -> (name=w203:string)  [unwired: 1 out]
          n32 = global read "[Global] Template.vi" "TemplateArray"() -> (w213:T34)
          n33 = Match Pattern(string=w203, regular expression=w205) -> (match substring=w206:string)  [unwired: 1 in, 3 out]
          n34 = Index Array(array=w213, index=w210) -> (element=w212:T35)
          n35 = Unbundle By Name(w212) -> ("TemplateArray"=w211:cluster{"ROI Name":string, "TemplateImage":T2}[])
          n36 = for {
            tunnel: w211 -> [w218] mode=indexing
            tunnel: w207 -> [w217]
            tunnel: [w215] -> w202
            stop <- w214 stop-if-true
            n37 = Unbundle(w218) -> ("ROI Name"=w216:string, "TemplateImage"=w215:T2)
            n38 = Wait (ms)(milliseconds to wait=u32 1) -> ()  [unwired: 1 out]
            n39 = Equal?(x=w217, y=w216) -> (x = y?=w214:bool)
          }
          n40 = Equal?(x=w206, y=w205) -> (x = y?=w204:bool)
          n41 = Select(t=w203, s=w204, f=w202) -> (s? t:f=w201:string)
        }
      }
      n42 = Unbundle By Name(w35) -> ("Reference System"=w34:T36, "Measurement System"=w33:T36)
      n43 = call "PatternMatch_MainFunction.vi"("ROI Descriptor"=w47, "Vision_Image In"=w43, "PatternMatchParameter"=w28) -> ("error out"=w44:errorcluster, "Number of Matches"=w32:i32, "Matches"=w57:T37[])  [unwired: 5 in, 1 out]
      n44 = case shown="No Error" w44 {
        tunnel: w57 -> [w84 _]
        tunnel: w56 -> [w83 _]
        tunnel: w55 -> [w82 _]
        tunnel: w34 -> [w81 _]
        tunnel: w33 -> [w80 _]
        tunnel: [w72 T14 {"numbers"=0, "results"=[]} ("PatternMatchResult")] -> w53
        tunnel: [w79 cluster{string, sgl, sgl}[] []] -> w52
        tunnel: w46 -> [w78 _]
        tunnel: w43 -> [w77 _]
        tunnel: w41 -> [w76 _]
        tunnel: [w75 _] -> w40
        tunnel: w32 -> [w73 _]
        frame No Error {
          n45 = for {
            tunnel: w83 -> [w148]
            tunnel: w82 -> [w147]
            tunnel: w84 -> [w150] mode=indexing
            tunnel: [w136] -> w74 mode=indexing
            tunnel: w81 -> [w132]
            tunnel: w80 -> [w133]
            tunnel: w78 -> [w127]
            tunnel: [w124] -> w79 mode=indexing
            tunnel: w77 -> [w121]
            tunnel: w76 -> [w97]
            tunnel: [w90] -> w75 mode=indexing
            i -> [w128]
            (unwired) 0.0 ("Rotation")
            n46 = Increment(x=w128) -> (x+1=w129:i32)
            n47 = Unbundle By Name(w150) -> ("Bounding Box"=w86:cluster{"x":sgl, "y":sgl}[], "Position.x"=w149:sgl, "Position.y"=w146:sgl, "Angle"=w88:sgl, "Score"=w135:sgl)
            n48 = Number To Decimal String(number=w129) -> (decimal integer string=w130:string)  [unwired: 1 in]
            n49 = for {
              tunnel: w86 -> [w162] mode=indexing
              tunnel: w148 -> [w164]
              tunnel: w147 -> [w163]
              tunnel: [w161] -> w85 mode=indexing
              n50 = Unbundle By Name(w162) -> ("x"=w166:sgl, "y"=w165:sgl)
              n51 = Add(x=w166, y=w164) -> (x+y=w159:sgl)
              n52 = Add(x=w165, y=w163) -> (x+y=w160:sgl)
              n53 = Bundle By Name(cluster=w162, "x"=w159, "y"=w160) -> (w161:cluster{"x":sgl, "y":sgl})
            }
            n54 = Concatenate Strings(w127, w130) -> (w91:string)
            n55 = Index Array(array=w85, index #1=0 ("index"), index #2=2 ("index")) -> (element #1=w145:cluster{"x":sgl, "y":sgl}, element #2=w144:cluster{"x":sgl, "y":sgl})
            n56 = Add(x=w149, y=w148) -> (x+y=w126:sgl)
            n57 = Unbundle(w145) -> ("x"=w143:sgl, "y"=w142:sgl)
            n58 = Unbundle(w144) -> ("x"=w141:sgl, "y"=w140:sgl)
            n59 = Add(x=w146, y=w147) -> (x+y=w125:sgl)
            n60 = Bundle("x"=w143, "y"=w142, "x"=w141, "y"=w140) -> ()  [unwired: 1 in, 1 out]
            n61 = Bundle(w126, w125) -> (w134:cluster{sgl, sgl})  [unwired: 1 in]
            n62 = call "overlaychange.vi"("Angle"=w88, "Bounding Box"=w85) -> ("OVERLAYRec"=w87:cluster{dbl, dbl, dbl, dbl, "Angle":dbl})  [unwired: 9 in]
            n63 = call "IMAQ Convert Rectangle to ROI"("Rectangle"=w87) -> ("ROI Descriptor"=w139:T12)  [unwired: 8 in, 1 out]
            n64 = call "IMAQ Convert Point to ROI"("Point"=w134) -> ("ROI Descriptor"=w89:T12)  [unwired: 8 in, 1 out]
            n65 = call "IMAQ TransformROI"("New Reference"=w133, "Base Reference"=w132, "ROI Descriptor"=w139) -> ("ROI Descriptor out"=w122:T12)  [unwired: 7 in, 1 out]
            n66 = call "IMAQ TransformROI"("New Reference"=w133, "Base Reference"=w132, "ROI Descriptor"=w89) -> ("ROI Descriptor out"=w131:T12)  [unwired: 7 in, 1 out]
            n67 = call "IMAQ Convert ROI to Point"("ROI Descriptor"=w131) -> ("Point"=w123:T15)  [unwired: 8 in, 1 out]
            n68 = call "IMAQ Convert ROI to Rectangle"("ROI Descriptor"=w122) -> ("Rectangle"=w120:T16)  [unwired: 8 in, 1 out]
            n69 = Unbundle(w120) -> ("Left"=w119:i32, "Top"=w118:i32, "Right"=w117:i32, "Bottom"=w116:i32)  [unwired: 1 out]
            n70 = Bundle("Right"=w117, "Bottom"=w116) -> (w114:cluster{"Right":i32, "Bottom":i32})  [unwired: 1 in]
            n71 = Bundle("Left"=w119, "Top"=w118) -> (w115:cluster{"Left":i32, "Top":i32})  [unwired: 1 in]
            n72 = call "IMAQ Convert Pixel to Real World"("Pixel Coordinates"=w123, "Calibrated Image"=w121) -> ("error out"=w100:errorcluster, "Real World Coordinates"=w96:cluster{"X":sgl, "Y":sgl})  [unwired: 4 in, 4 out]
            n73 = Build Array(w115, w114) -> (w113:cluster{"Right":i32, "Bottom":i32}[])
            n74 = call "IMAQ Convert Pixel to Real World"("Array of Pixel Coordinates"=w113, "Calibrated Image"=w121) -> ("error out"=w99:errorcluster, "Array of Real World Coordinates"=w112:cluster{"X":sgl, "Y":sgl}[])  [unwired: 4 in, 4 out]
            n75 = Merge Errors(w100, w99) -> (w98:errorcluster)
            n76 = call <vilib>:"Clear Errors.vi"("error in (no error)"=w98) -> ()  [unwired: 5 in, 2 out]
            n77 = Index Array(array=w112, index #1=0 ("index"), index #2=1 ("index")) -> (element #1=w109:cluster{"X":sgl, "Y":sgl}, element #2=w108:cluster{"X":sgl, "Y":sgl})
            n78 = Unbundle(w123) -> ("X"=w93:sgl, "Y"=w92:sgl)
            n79 = Unbundle(w96) -> ("X"=w95:sgl, "Y"=w94:sgl)
            n80 = Unbundle(w108) -> ("X"=w105:sgl, "Y"=w104:sgl)
            n81 = Unbundle(w109) -> ("X"=w107:sgl, "Y"=w106:sgl)
            n82 = Bundle(cluster=T16 {"Left"=0, "Top"=0, "Right"=0, "Bottom"=0, "Rotation"=0.0} ("Rectangle"), "Left"=w107, "Top"=w106, "Right"=w105, "Bottom"=w104, "Rotation"=0.0) -> (w101:T16)
            n83 = Bundle("ROI Descriptor out"=w122, "Point"=w123, "Angle"=w88, "Score"=w135, "Real World Coordinates"=w96, "Rectangle"=w101) -> (w136:T38)  [unwired: 1 in]
            n84 = Bundle(w91, "X"=w93, "Y"=w92) -> (w90:cluster{string, "X":sgl, "Y":sgl})  [unwired: 1 in]
            n85 = case shown="False" w97 {
              tunnel: w91 -> [w154 w158]
              tunnel: [w153 w155] -> w124
              tunnel: w93 -> [w152 _]
              tunnel: w92 -> [w151 _]
              tunnel: w95 -> [_ w157]
              tunnel: w94 -> [_ w156]
              frame False {
                n86 = Bundle(w154, "X"=w152, "Y"=w151) -> (w153:cluster{string, "X":sgl, "Y":sgl})  [unwired: 1 in]
              }
              frame True {
                n87 = Bundle(w158, "X"=w157, "Y"=w156) -> (w155:cluster{string, "X":sgl, "Y":sgl})  [unwired: 1 in]
              }
            }
          }
          n88 = Bundle(cluster=T14 {"numbers"=0, "results"=[]} ("PatternMatchResult"), "numbers"=w73, "results"=w74) -> (w72:T14)
        }
        frame Error {
        }
      }
      n89 = disable-structure shown="Enabled" {
        disable-tunnel: w44 -> [w221 w222]
        disable-tunnel: w47 -> [w220 _]
        disable-tunnel: [_ w222] -> w45
        frame Disabled {
          n90 = call "Imaq Dispose"("Image"=w220, "error in (no error)"=w221) -> ()  [unwired: 4 in, 1 out]
        }
        frame Enabled {
        }
      }
      n91 = To Variant(anything=w53) -> (Variant=w54:variant)
    }
    frame 2 {
      w234 = "_" ("string")
      w247 = T39 {"Edge Options"={"Edge Polarity"=0, "Kernel Size"=3, "Width"=5, "Minimum Edge Strength"=10.0, "Interpolation Type"=1, "Data Processing Method"=0}, "Process"=2, "Number of Matches Requested"=1, "ROI Descriptor"={"Global Rectangle"=[], "Contours"=[]}}  # Analysis_Edge Detection_Parameter
      n92 = Concatenate Strings(w230, w234, w233, w234, "Edge" ("string")) -> (w232:string)
      n93 = Variant To Data(type=w247, Variant=w248) -> (data=w246:T39)  [unwired: 1 in, 1 out]
      n94 = Unbundle By Name(w246) -> ("Edge Options"=w245:T40, "Process"=w244:u16, "Number of Matches Requested"=w243:i32, "ROI Descriptor"=w225:T41)
      n95 = call "Edge Detection_Main Function.vi"("Refnum in"=w249, "Process"=w244, "Edge Options"=w245, "Number of Matches Requested IN"=w243, "ROI"=w225, "error in (no error)"=w229) -> ("Image Out"=w226:T2, "Edge Information"=w241:T17[], "Number of Edges Detected"=w240:i32, "error out"=w228:errorcluster)  [unwired: 6 in]
      n96 = Bundle("Edge Information"=w241, "Number of Edges Detected"=w240) -> (w237:T18)  [unwired: 1 in]
      n97 = case shown="No Error" w228 {
        tunnel: w239 -> [w263 _]
        tunnel: w238 -> [w262 _]
        tunnel: w237 -> [w256 _]
        tunnel: [w253 T18 {"Edge Information"=[], "Number of Edges Detected"=0} ("output cluster")] -> w236
        tunnel: w232 -> [w261 _]
        tunnel: [w260 cluster{string, sgl, sgl}[] []] -> w231
        tunnel: w227 -> [w259 _]
        tunnel: w226 -> [w255 _]
        tunnel: w225 -> [w252 _]
        tunnel: w224 -> [w251 _]
        tunnel: [w250 _] -> w223
        frame No Error {
          n98 = Unbundle By Name(w256) -> ("Edge Information"=w265:T17[], "Number of Edges Detected"=w264:i32)
          n99 = Unbundle By Name(w259) -> ("Reference System"=w258:T36, "Measurement System"=w257:T36)
          n100 = for {
            N: w264 -> [_]
            tunnel: w265 -> [w300] mode=indexing
            tunnel: w263 -> [w288]
            tunnel: w262 -> [w286]
            tunnel: w261 -> [w307]
            tunnel: [w306] -> w260 mode=indexing
            tunnel: w258 -> [w303]
            tunnel: w257 -> [w302]
            tunnel: w255 -> [w299]
            tunnel: [w298] -> w254 mode=indexing
            tunnel: w252 -> [w294]
            tunnel: w251 -> [w279]
            tunnel: [w272] -> w250 mode=indexing
            i -> [w308]
            n101 = Unbundle By Name(w294) -> ("Contours"=w293:T42)
            n102 = Unbundle By Name(w300) -> ("Location (Pixel)"=w311:cluster{"X":sgl, "Y":sgl})
            n103 = Increment(x=w308) -> (x+1=w309:i32)
            n104 = Index Array(array=w293) -> (element=w292:T43)  [unwired: 1 in]
            n105 = Number To Decimal String(number=w309) -> (decimal integer string=w310:string)  [unwired: 1 in]
            n106 = Unbundle By Name(w292) -> ("Points"=w291:i32[])
            n107 = Unbundle By Name(w311) -> ("X"=w313:sgl, "Y"=w312:sgl)
            n108 = Concatenate Strings(w307, w310) -> (w275:string)
            n109 = Index Array(array=w291, index #1=0 ("index"), index #2=1 ("index")) -> (element #1=w287:i32, element #2=w285:i32)
            n110 = Add(x=w313, y=w288) -> (x+y=w274:sgl)
            n111 = Add(x=w312, y=w286) -> (x+y=w273:sgl)
            n112 = Bundle By Name(cluster=w311, "X"=w274, "Y"=w273) -> (w305:cluster{"X":sgl, "Y":sgl})
            n113 = Add(x=w288, y=w287) -> (x+y=w283:i32)
            n114 = Add(x=w286, y=w285) -> (x+y=w284:i32)
            n115 = call "IMAQ Convert Point to ROI"("Point"=w305) -> ("ROI Descriptor"=w304:T12)  [unwired: 8 in, 1 out]
            n116 = Bundle(w283, w284) -> (w295:cluster{i32, i32})  [unwired: 1 in]
            n117 = call "IMAQ TransformROI"("New Reference"=w302, "Base Reference"=w303, "ROI Descriptor"=w304) -> ("ROI Descriptor out"=w301:T12)  [unwired: 7 in, 1 out]
            n118 = call "IMAQ Convert ROI to Point"("ROI Descriptor"=w301) -> ("Point"=w268:T15)  [unwired: 8 in, 1 out]
            n119 = Build Array(w295, w268) -> (w271:T15[])
            n120 = Unbundle(w268) -> ("X"=w267:sgl, "Y"=w266:sgl)
            n121 = call "IMAQ Convert Pixel to Real World"("Array of Pixel Coordinates"=w271, "Calibrated Image"=w299) -> ("error out"=w270:errorcluster, "Array of Real World Coordinates"=w282:cluster{"X":sgl, "Y":sgl}[])  [unwired: 4 in, 4 out]
            n122 = Index Array(array=w282, index #1=0 ("index"), index #2=1 ("index")) -> (element #2=w278:cluster{"X":sgl, "Y":sgl})  [unwired: 1 out]
            n123 = call "IMAQ Point Distances"("Points"=w282, "error in (no error)"=w270) -> ("Distances"=w281:sgl[], "error out"=w269:errorcluster)  [unwired: 3 in]
            n124 = Unbundle(w278) -> ("X"=w277:sgl, "Y"=w276:sgl)
            n125 = call <vilib>:"Clear Errors.vi"("error in (no error)"=w269) -> ()  [unwired: 5 in, 2 out]
            n126 = Index Array(array=w281) -> (element=w280:sgl)  [unwired: 1 in]
            n127 = Bundle(w275, "X"=w267, "Y"=w266) -> (w272:cluster{string, "X":sgl, "Y":sgl})  [unwired: 1 in]
            n128 = Bundle By Name(cluster=w300, "Location (Pixel)"=w268, "Location (Real-World)"=w278, "Distance (Real-World)"=w280) -> (w298:T17)
            n129 = case shown="True" w279 {
              tunnel: w274 -> [w317 _]
              tunnel: w273 -> [w316 _]
              tunnel: w275 -> [w315 w321]
              tunnel: [w314 w318] -> w306
              tunnel: w277 -> [_ w320]
              tunnel: w276 -> [_ w319]
              frame False {
                n130 = Bundle(w315, w317, w316) -> (w314:cluster{string, sgl, sgl})  [unwired: 1 in]
              }
              frame True {
                n131 = Bundle(w321, "X"=w320, "Y"=w319) -> (w318:cluster{string, "X":sgl, "Y":sgl})  [unwired: 1 in]
              }
            }
          }
          n132 = Bundle By Name(cluster=w256, "Edge Information"=w254) -> (w253:T18)
        }
        frame Error {
        }
      }
      n133 = To Variant(anything=w236) -> (Variant=w242:variant)
    }
    frame 3 {
      w330 = "_" ("string")
      w336 = string[] ["", "Codabar", "Code39", "Code93", "Code128", "EAN8", "EAN13"]  # Barcode type strings
      w345 = T44 {"Barcode Search Options"={"Min Bar Width"=0.0, "Min Edge Strength"=0.0, "Min Bars"=0.0, "Skip Location Search?"=FALSE}, "Barcode Types To Search"=[enum."EAN 13", enum."Code 128", enum."Code 39"], "Barcode Grading Options"={"Calculate Grading Report"=FALSE, "Scan Width "=0.0}, "Number of Matches Requested"=1, "ROI"={"Global Rectangle"=[], "Contours"=[]}}  # Analysis_Barcode 1D_Parameter
      n134 = Concatenate Strings(w327, w330, w328, w330, "Barcode 1D" ("string")) -> ()  [unwired: 1 out]
      n135 = Variant To Data(type=w345, Variant=w346) -> (data=w344:T44)  [unwired: 1 in, 1 out]
      n136 = Unbundle By Name(w344) -> ("Barcode Search Options"=w340:T45, "Barcode Types To Search"=w341:T46, "Barcode Grading Options"=w339:T47, "Number of Matches Requested"=w343:i32, "ROI"=w338:T41)
      n137 = call "Barcode 1D_Main Function.vi"("Refnum in"=w342, "Barcode type strings IN"=w336, "Number of Matches Requested IN"=w343, "Barcode Search Options IN"=w340, "Barcode Types To Search IN"=w341, "error in (no error)"=w326, "Barcode Grading Options IN"=w339, "ROI Descriptor"=w338) -> ("Refnum out"=w337:T2, "Barcodes"=w335:T48, "error out"=w325:errorcluster)  [unwired: 3 in, 2 out]
      n138 = case shown="No Error" w325 {
        tunnel: w336 -> [w354 _]
        tunnel: w335 -> [w353 _]
        tunnel: [w350 T19 {[], [], "Barcodes"=[]}] -> w334
        tunnel: w332 -> [w349 _]
        tunnel: w331 -> [w348 _]
        tunnel: w324 -> [w347 _]
        frame No Error {
          n139 = for {
            tunnel: w353 -> [w373] mode=indexing
            tunnel: w354 -> [w372]
            tunnel: [w369] -> _ mode=indexing
            tunnel: w349 -> [w360]
            tunnel: w348 -> [w361]
            tunnel: [w359] -> w351 mode=indexing
            tunnel: [w358] -> w352 mode=indexing
            tunnel: w347 -> [w357]
            n140 = Unbundle By Name(w357) -> ("Reference System"=w356:T36, "Measurement System"=w355:T36)
            n141 = Unbundle By Name(w373) -> ("Bounding Box"=w362:cluster{"x":sgl, "y":sgl}[], "Barcode Type"=w370:u32, "Special Char 1"=w367:string, "Special Char 2"=w366:string, "Data"=w365:string, "Checksum(s)"=w364:string)
            n142 = for {
              tunnel: w362 -> [w381] mode=indexing
              tunnel: w360 -> [w384]
              tunnel: w361 -> [w383]
              tunnel: [w374] -> w359 mode=indexing
              tunnel: w356 -> [w379]
              tunnel: w355 -> [w378]
              n143 = Unbundle By Name(w381) -> ("x"=w386:sgl, "y"=w385:sgl)
              n144 = Add(x=w386, y=w384) -> (x+y=w382:sgl)
              n145 = Add(x=w385, y=w383) -> (x+y=w380:sgl)
              n146 = Bundle By Name(cluster=w381, "x"=w382, "y"=w380) -> (w377:cluster{"x":sgl, "y":sgl})
              n147 = call "IMAQ Convert Point to ROI"("Point"=w377) -> ("ROI Descriptor"=w376:T12)  [unwired: 8 in, 1 out]
              n148 = call "IMAQ TransformROI"("New Reference"=w378, "Base Reference"=w379, "ROI Descriptor"=w376) -> ("ROI Descriptor out"=w375:T12)  [unwired: 7 in, 1 out]
              n149 = call "IMAQ Convert ROI to Point"("ROI Descriptor"=w375) -> ("Point"=w374:T15)  [unwired: 8 in, 1 out]
            }
            n150 = Index Array(array=w372, index=w370) -> (element=w368:string)
            n151 = Concatenate Strings(w368, ": " ("string"), w367, w366, w365, w364) -> (w358:string)
            n152 = Concatenate Strings(w367, w366, w365, w364) -> (w363:string)
            n153 = Bundle(w363, w368) -> (w369:cluster{string, string})  [unwired: 1 in]
          }
          n154 = Bundle(w351, w352, "Barcodes"=w353) -> (w350:T49)  [unwired: 1 in]
        }
        frame Error {
        }
      }
      n155 = To Variant(anything=w334) -> (Variant=w333:variant)
    }
    frame 4 {
      w402 = T50 {"ROI"={"Global Rectangle"=[], "Contours"=[]}, "Barcode Type"=enum."PDF417", "Data Matrix Parameter"={"Data Matrix Description Options"={"Aspect Ratio"=0.0, "Rows"=0, "Columns"=0, "Rectangle"=FALSE, "ECC"=-2, "Barcode Polarity"=0, "Cell Fill Percentage"=-2, "Minimum Border Integrity %"=80.0, "Mirror Mode"=-2}, "Data Matrix Search Options"={"Rotation Mode"=enum."Unlimited", "Skip Location?"=FALSE, "Edge Threshold"=30, "Demodulation Mode"=-2, "Cell Sample Size"=-2, "Cell Filter Mode"=-2, "Skew Degrees Allowed"=5, "Maximum Iterations"=500, "Initial Search Vector Width"=5}, "Data Matrix Size Options"={"Data Matrix Size"={"Minimum Size"=0, "Maximum Size"=0}, "Quiet Zone Width"=10}, "Advanced Options"=[]}, "PDF147 Search Mode"=enum."Multiple Barcodes", "QR Code Parameter"={"QR Search Options"={"Rotation Mode"=enum."Unlimited", "Skip Location?"=FALSE, "Edge Threshold"=30, "Demodulation Mode"=-2, "Cell Sample Size"=-2, "Cell Filter Mode"=-2, "Skew Degrees Allowed"=5}, "QR Description Options"={"Matrix Size (cells)"=0, "Barcode Polarity"=-2, "Mirror Mode"=-2, "QR Model"=0}, "QR Code Cell Size (pixels)"={"Minimum Size"=3, "Maximum Size"=7}}}  # Analysis_Barcode 2D_Parameter
      n156 = Variant To Data(type=w402, Variant=w403) -> (data=w389:T50, error out=w388:errorcluster)  [unwired: 1 in]
      n157 = call <vilib>:"Clear Errors.vi"("error in (no error)"=w388) -> ()  [unwired: 5 in, 2 out]
      n158 = call "Barcode 2D_Main Function.vi"("error in (no error)"=w392, "2D Barcode Parameter in"=w389, "Image In"=w401) -> ("error out"=w391:errorcluster, "Bounding Box"=w399:cluster{"x":sgl, "y":sgl}[], "Data"=w400:string, "Image Out"=w397:T2)  [unwired: 5 in]
      n159 = Bundle("Data"=w400, "Bounding Box"=w399) -> (w396:T66)  [unwired: 1 in]
      n160 = case shown="No Error" w391 {
        tunnel: w396 -> [w412 _]
        tunnel: [w410 T20 {"Data"="", []}] -> w395
        tunnel: w394 -> [w408 _]
        tunnel: w393 -> [w407 _]
        tunnel: w390 -> [w406 _]
        frame No Error {
          n161 = Unbundle By Name(w412) -> ("Data"=w409:string, "Bounding Box"=w413:cluster{"x":sgl, "y":sgl}[])
          n162 = Unbundle By Name(w406) -> ("Reference System"=w405:T36, "Measurement System"=w404:T36)
          n163 = for {
            tunnel: w413 -> [w421] mode=indexing
            tunnel: w408 -> [w424]
            tunnel: w407 -> [w423]
            tunnel: [w414] -> w411 mode=indexing
            tunnel: w405 -> [w417]
            tunnel: w404 -> [w416]
            n164 = Unbundle By Name(w421) -> ("x"=w426:sgl, "y"=w425:sgl)
            n165 = Add(x=w426, y=w424) -> (x+y=w422:sgl)
            n166 = Add(x=w425, y=w423) -> (x+y=w420:sgl)
            n167 = Bundle By Name(cluster=w421, "x"=w422, "y"=w420) -> (w419:cluster{"x":sgl, "y":sgl})
            n168 = call "IMAQ Convert Point to ROI"("Point"=w419) -> ("ROI Descriptor"=w418:T12)  [unwired: 8 in, 1 out]
            n169 = call "IMAQ TransformROI"("New Reference"=w416, "Base Reference"=w417, "ROI Descriptor"=w418) -> ("ROI Descriptor out"=w415:T12)  [unwired: 7 in, 1 out]
            n170 = call "IMAQ Convert ROI to Point"("ROI Descriptor"=w415) -> ("Point"=w414:T15)  [unwired: 8 in, 1 out]
          }
          n171 = Bundle("Data"=w409, w411) -> (w410:cluster{"Data":string, T15[]})  [unwired: 1 in]
        }
        frame Error {
        }
      }
      n172 = To Variant(anything=w395) -> (Variant=w398:variant)
    }
    frame 5 {
      w434 = "_" ("string")
      w455 = T67 {"Clamp Settings"={"Contrast"=40, "Filter width"=4, "Steepness"=2, "Subsampling Ratio"=5, "Show Search Area"=TRUE, "Show Search Lines"=TRUE, "Show Edges Found"=TRUE, "Show Result"=TRUE}, "ROI Descriptor"={"Global Rectangle"=[498, 111, 1545, 770], "Contours"=[{"Contour Type"=0, "ROI Type"=12, "Points"=[498, 111, 1545, 770, 0]}]}, "Process"=0}  # Analysis_Clamp_Parameter
      n173 = Variant To Data(type=w455, Variant=w456) -> (data=w454:T67)  [unwired: 1 in, 1 out]
      n174 = Unbundle By Name(w454) -> ("Clamp Settings"=w441:T68, "ROI Descriptor"=w440:T41, "Process"=w452:u16)
      n175 = Concatenate Strings(w433, w434, w432, w434, "Clamp" ("string")) -> (w431:string)
      n176 = call "Clamp_Main Function.vi"("Refnum in"=w437, "Clamp Settings"=w441, "ROI"=w440, "error in (no error)"=w439, "Process In"=w452) -> ("Line Coordinates"=w449:T69, "appended array"=w447:cluster{"X":sgl, "Y":sgl}[], "Perpendicular Lines"=w450:T69, "Points"=w448:cluster{"X":sgl, "Y":sgl}[], "Refnum out"=w451:T2, "Distance"=w443:sgl, "Edge Coordinates"=w442:cluster{"X":sgl, "Y":sgl}[], "error out"=w436:errorcluster)  [unwired: 7 in]
      n177 = case shown="No Error" w436 {
        tunnel: w450 -> [w493 _]
        tunnel: w449 -> [w492 _]
        tunnel: w448 -> [w491 _]
        tunnel: w447 -> [w490 _]
        tunnel: w446 -> [w478 _]
        tunnel: w445 -> [w477 _]
        tunnel: [w489 T21 {"Points"=[], "Perpendicular Lines"=[], "appended array"=[], "Line Coordinates"=[], "Clamp Settings"={"Contrast"=0, "Filter width"=0, "Steepness"=0, "Subsampling Ratio"=0, "Show Search Area"=FALSE, "Show Search Lines"=FALSE, "Show Edges Found"=FALSE, "Show Result"=FALSE}, "ROI Descriptor"={"Global Rectangle"=[], "Contours"=[]}, "Distance"=0.0, "Edge Coordinates"=[{"X"=441.67966, "Y"=663.0}, {"X"=684.4586, "Y"=655.0}], "Edge Coordinates  (Real World)"=[{"X"=441.67966, "Y"=663.0}, {"X"=684.4586, "Y"=655.0}], "Distance (Real World)"=0.0} ("Cluster")] -> w444
        tunnel: w443 -> [w460 _]
        tunnel: w442 -> [w481 _]
        tunnel: w441 -> [w487 _]
        tunnel: w440 -> [w486 _]
        tunnel: w438 -> [w485 _]
        tunnel: w437 -> [w483 _]
        tunnel: w431 -> [w473 _]
        tunnel: w430 -> [w476 _]
        tunnel: [w474 _] -> w429
        tunnel: [w475 _] -> w428
        frame No Error {
          n178 = Unbundle By Name(w485) -> ("Reference System"=w480:T36, "Measurement System"=w479:T36)
          n179 = for {
            tunnel: w491 -> [w539] mode=indexing
            tunnel: w478 -> [w541]
            tunnel: w477 -> [w540]
            tunnel: [w531] -> w461 mode=indexing
            tunnel: w480 -> [w536]
            tunnel: w479 -> [w535]
            n180 = Unbundle By Name(w539) -> ("X"=w543:sgl, "Y"=w542:sgl)
            n181 = Add(x=w542, y=w540) -> (x+y=w537:sgl)
            n182 = Add(x=w543, y=w541) -> (x+y=w538:sgl)
            n183 = Bundle By Name(cluster=w539, "X"=w538, "Y"=w537) -> (w534:cluster{"X":sgl, "Y":sgl})
            n184 = call "IMAQ Convert Point to ROI"("Point"=w534) -> ("ROI Descriptor"=w533:T12)  [unwired: 8 in, 1 out]
            n185 = call "IMAQ TransformROI"("New Reference"=w535, "Base Reference"=w536, "ROI Descriptor"=w533) -> ("ROI Descriptor out"=w532:T12)  [unwired: 7 in, 1 out]
            n186 = call "IMAQ Convert ROI to Point"("ROI Descriptor"=w532) -> ("Point"=w531:T15)  [unwired: 8 in, 1 out]
          }
          n187 = for {
            tunnel: w493 -> [w591] mode=indexing
            tunnel: w478 -> [w579]
            tunnel: w477 -> [w578]
            tunnel: [w580] -> w459 mode=indexing
            tunnel: w480 -> [w573]
            tunnel: w479 -> [w572]
            n188 = Unbundle(w591) -> (w590:cluster{"X":sgl, "Y":sgl}, w589:cluster{"X":sgl, "Y":sgl})
            n189 = Unbundle(w590) -> ("X"=w588:sgl, "Y"=w587:sgl)
            n190 = Unbundle(w589) -> ("X"=w586:sgl, "Y"=w585:sgl)
            n191 = Add(x=w588, y=w579) -> (x+y=w584:sgl)
            n192 = Add(x=w587, y=w578) -> (x+y=w583:sgl)
            n193 = Add(x=w586, y=w579) -> (x+y=w582:sgl)
            n194 = Add(x=w585, y=w578) -> (x+y=w581:sgl)
            n195 = Bundle(w584, w583) -> (w577:cluster{sgl, sgl})  [unwired: 1 in]
            n196 = Bundle(w582, w581) -> (w576:cluster{sgl, sgl})  [unwired: 1 in]
            n197 = call "IMAQ Convert Point to ROI"("Point"=w577) -> ("ROI Descriptor"=w574:T12)  [unwired: 8 in, 1 out]
            n198 = call "IMAQ Convert Point to ROI"("Point"=w576) -> ("ROI Descriptor"=w575:T12)  [unwired: 8 in, 1 out]
            n199 = call "IMAQ TransformROI"("New Reference"=w572, "Base Reference"=w573, "ROI Descriptor"=w575) -> ("ROI Descriptor out"=w569:T12)  [unwired: 7 in, 1 out]
            n200 = call "IMAQ TransformROI"("New Reference"=w572, "Base Reference"=w573, "ROI Descriptor"=w574) -> ("ROI Descriptor out"=w571:T12)  [unwired: 7 in, 1 out]
            n201 = call "IMAQ Convert ROI to Point"("ROI Descriptor"=w571) -> ("Point"=w570:T15)  [unwired: 8 in, 1 out]
            n202 = call "IMAQ Convert ROI to Point"("ROI Descriptor"=w569) -> ("Point"=w568:T15)  [unwired: 8 in, 1 out]
            n203 = Bundle("Point"=w570, "Point"=w568) -> (w580:cluster{"Point":T15, "Point":T15})  [unwired: 1 in]
          }
          n204 = for {
            tunnel: w490 -> [w526] mode=indexing
            tunnel: w478 -> [w528]
            tunnel: w477 -> [w527]
            tunnel: [w518] -> w457 mode=indexing
            tunnel: w480 -> [w522]
            tunnel: w479 -> [w521]
            n205 = Unbundle By Name(w526) -> ("X"=w530:sgl, "Y"=w529:sgl)
            n206 = Add(x=w529, y=w527) -> (x+y=w524:sgl)
            n207 = Add(x=w530, y=w528) -> (x+y=w525:sgl)
            n208 = Bundle By Name(cluster=w526, "X"=w525, "Y"=w524) -> (w523:cluster{"X":sgl, "Y":sgl})
            n209 = call "IMAQ Convert Point to ROI"("Point"=w523) -> ("ROI Descriptor"=w520:T12)  [unwired: 8 in, 1 out]
            n210 = call "IMAQ TransformROI"("New Reference"=w521, "Base Reference"=w522, "ROI Descriptor"=w520) -> ("ROI Descriptor out"=w519:T12)  [unwired: 7 in, 1 out]
            n211 = call "IMAQ Convert ROI to Point"("ROI Descriptor"=w519) -> ("Point"=w518:T15)  [unwired: 8 in, 1 out]
          }
          n212 = for {
            tunnel: w481 -> [w513] mode=indexing
            tunnel: w478 -> [w515]
            tunnel: w477 -> [w514]
            tunnel: [w506] -> w458 mode=indexing
            tunnel: w480 -> [w512]
            tunnel: w479 -> [w508]
            tunnel: w473 -> [w507]
            tunnel: [w503] -> w474 mode=indexing
            n213 = Unbundle By Name(w513) -> ("X"=w517:sgl, "Y"=w516:sgl)
            n214 = Add(x=w516, y=w514) -> (x+y=w504:sgl)
            n215 = Add(x=w517, y=w515) -> (x+y=w505:sgl)
            n216 = Bundle By Name(cluster=w513, "X"=w505, "Y"=w504) -> (w511:cluster{"X":sgl, "Y":sgl})
            n217 = call "IMAQ Convert Point to ROI"("Point"=w511) -> ("ROI Descriptor"=w510:T12)  [unwired: 8 in, 1 out]
            n218 = call "IMAQ TransformROI"("New Reference"=w508, "Base Reference"=w512, "ROI Descriptor"=w510) -> ("ROI Descriptor out"=w509:T12)  [unwired: 7 in, 1 out]
            n219 = call "IMAQ Convert ROI to Point"("ROI Descriptor"=w509) -> ("Point"=w506:T15)  [unwired: 8 in, 1 out]
            n220 = Bundle(w507, w505, w504) -> (w503:cluster{string, sgl, sgl})  [unwired: 1 in]
          }
          n221 = for {
            tunnel: w492 -> [w544] mode=indexing
            tunnel: [w557] -> w488 mode=indexing
            tunnel: w478 -> [w556]
            tunnel: w477 -> [w555]
            tunnel: w480 -> [w551]
            tunnel: w479 -> [w549]
            n222 = Unbundle(w544) -> (w567:cluster{"X":sgl, "Y":sgl}, w566:cluster{"X":sgl, "Y":sgl})
            n223 = Unbundle(w567) -> ("X"=w565:sgl, "Y"=w564:sgl)
            n224 = Unbundle(w566) -> ("X"=w563:sgl, "Y"=w562:sgl)
            n225 = Add(x=w565, y=w556) -> (x+y=w561:sgl)
            n226 = Add(x=w564, y=w555) -> (x+y=w560:sgl)
            n227 = Add(x=w563, y=w556) -> (x+y=w559:sgl)
            n228 = Add(x=w562, y=w555) -> (x+y=w558:sgl)
            n229 = Bundle(w561, w560) -> (w554:cluster{sgl, sgl})  [unwired: 1 in]
            n230 = Bundle(w559, w558) -> (w553:cluster{sgl, sgl})  [unwired: 1 in]
            n231 = call "IMAQ Convert Point to ROI"("Point"=w553) -> ("ROI Descriptor"=w550:T12)  [unwired: 8 in, 1 out]
            n232 = call "IMAQ Convert Point to ROI"("Point"=w554) -> ("ROI Descriptor"=w552:T12)  [unwired: 8 in, 1 out]
            n233 = call "IMAQ TransformROI"("New Reference"=w549, "Base Reference"=w551, "ROI Descriptor"=w552) -> ("ROI Descriptor out"=w548:T12)  [unwired: 7 in, 1 out]
            n234 = call "IMAQ TransformROI"("New Reference"=w549, "Base Reference"=w551, "ROI Descriptor"=w550) -> ("ROI Descriptor out"=w546:T12)  [unwired: 7 in, 1 out]
            n235 = call "IMAQ Convert ROI to Point"("ROI Descriptor"=w548) -> ("Point"=w547:T15)  [unwired: 8 in, 1 out]
            n236 = call "IMAQ Convert ROI to Point"("ROI Descriptor"=w546) -> ("Point"=w545:T15)  [unwired: 8 in, 1 out]
            n237 = Bundle("Point"=w547, "Point"=w545) -> (w557:cluster{"Point":T15, "Point":T15})  [unwired: 1 in]
          }
          n238 = call "IMAQ Convert Pixel to Real World"("Array of Pixel Coordinates"=w458, "Calibrated Image"=w483) -> ("error out"=w463:errorcluster, "Array of Real World Coordinates"=w472:cluster{"X":sgl, "Y":sgl}[])  [unwired: 4 in, 4 out]
          n239 = Index Array(array=w472) -> (element #1=w466:cluster{"X":sgl, "Y":sgl}, element #2=w468:cluster{"X":sgl, "Y":sgl})  [unwired: 2 in]
          n240 = Unbundle By Name(w466) -> ("X"=w471:sgl)
          n241 = Unbundle By Name(w468) -> ("Y"=w470:sgl)
          n242 = Bundle("X"=w471, "Y"=w470) -> (w469:cluster{"X":sgl, "Y":sgl})  [unwired: 1 in]
          n243 = Bundle(w469, w468) -> (w467:T22)  [unwired: 1 in]
          n244 = call "IMAQ Perpendicular Line"("error in (no error)"=w463, "Point"=w466, "Line"=w467) -> ("error out"=w462:errorcluster, "Distance"=w465:dbl)  [unwired: 6 in, 1 out]
          n245 = Build Array(w465) -> (w464:dbl[])
          n246 = Index Array(array=w464) -> (element=w482:dbl)  [unwired: 1 in]
          n247 = call <vilib>:"Clear Errors.vi"("error in (no error)"=w462) -> ()  [unwired: 5 in, 2 out]
          n248 = Bundle By Name(cluster=T21 {"Points"=[], "Perpendicular Lines"=[], "appended array"=[], "Line Coordinates"=[], "Clamp Settings"={"Contrast"=0, "Filter width"=0, "Steepness"=0, "Subsampling Ratio"=0, "Show Search Area"=FALSE, "Show Search Lines"=FALSE, "Show Edges Found"=FALSE, "Show Result"=FALSE}, "ROI Descriptor"={"Global Rectangle"=[], "Contours"=[]}, "Distance"=0.0, "Edge Coordinates"=[{"X"=441.67966, "Y"=663.0}, {"X"=684.4586, "Y"=655.0}], "Edge Coordinates  (Real World)"=[{"X"=441.67966, "Y"=663.0}, {"X"=684.4586, "Y"=655.0}], "Distance (Real World)"=0.0} ("Cluster"), "Points"=w461, "Perpendicular Lines"=w459, "appended array"=w457, "Line Coordinates"=w488, "Edge Coordinates"=w458, "Distance"=w460, "Clamp Settings"=w487, "ROI Descriptor"=w486, "Edge Coordinates  (Real World)"=w472, "Distance (Real World)"=w482) -> (w489:T21)
          n249 = case shown="False" w476 {
            tunnel: [w494 w495] -> w475
            tunnel: w474 -> [w494 _]
            tunnel: w472 -> [_ w497]
            tunnel: w473 -> [_ w496]
            frame False {
            }
            frame True {
              n250 = for {
                tunnel: w497 -> [w501] mode=indexing
                tunnel: w496 -> [w502]
                tunnel: [w498] -> w495 mode=indexing
                n251 = Unbundle(w501) -> ("X"=w500:sgl, "Y"=w499:sgl)
                n252 = Bundle(w502, "X"=w500, "Y"=w499) -> (w498:cluster{string, "X":sgl, "Y":sgl})  [unwired: 1 in]
              }
            }
          }
        }
        frame Error {
        }
      }
      n253 = To Variant(anything=w444) -> (Variant=w453:variant)
    }
    frame 6 {
      w599 = "_" ("string")
      w620 = T70 {"Overlay Settings"={"Show Search Area"=FALSE, "Show Curves"=FALSE, "Show Clamp Locations"=FALSE, "Show Result"=FALSE, "Search Area Color"=0, "Curves Color"=0, "Clamp Locations Color"=0, "Result Color"=0, "Overlay Group Name"=""}, "Curve Extraction Settings"={"Extraction Mode"=0, "Edge Threshold"=0, "Edge Filter Size"=0, "Min Length"=0, "Row Search Step Size"=0, "Col Search Step Size"=0, "Max Endpoint Gap"=0, "Closed"=FALSE, "Subpixel"=FALSE}, "Clamp Settings"={"Angle Range (+/-)"=0.0, "Edge Polarity"={"Start"=0, "End"=0}}, "ROI"={"Global Rectangle"=[], "Contours"=[]}}  # Analysis_Clamp MAX_Parameter
      n254 = Variant To Data(type=w620, Variant=w622) -> (data=w619:T70)  [unwired: 1 in, 1 out]
      n255 = Unbundle By Name(w619) -> ("Overlay Settings"=w618:T71, "Curve Extraction Settings"=w617:T72, "Clamp Settings"=w616:T73, "ROI"=w613:T41)
      n256 = Concatenate Strings(w598, w599, w597, w599, "Clmap Max" ("string")) -> (w596:string)
      n257 = call "Clamp MAX_Main Function.vi"("Refnum in"=w621, "ROI"=w613, "error in (no error)"=w609, "Clamp Settings in"=w616, "Curve Extraction Settings in"=w617, "Overlay Settings"=w618) -> ("error out"=w608:errorcluster, "Clamp Points"=w614:T74, "Clamp Results"=w615:T75, "Refnum out"=w606:T2)  [unwired: 2 in]
      n258 = Bundle("Clamp Results"=w615, "Clamp Points"=w614) -> (w605:T76)  [unwired: 1 in]
      n259 = case shown="No Error" w608 {
        tunnel: w612 -> [w661 _]
        tunnel: w611 -> [w660 _]
        tunnel: w605 -> [w659 _]
        tunnel: w607 -> [w658 _]
        tunnel: w606 -> [w643 _]
        tunnel: [w640 cluster{"Point":T15, "Point":T15} {"Point"={"X"=0.0, "Y"=0.0}, "Point"={"X"=0.0, "Y"=0.0}}] -> w604
        tunnel: [w638 sgl 0.0] -> w603
        tunnel: [w632 T22 {{"X"=0.0, "Y"=0.0}, {"X"=0.0, "Y"=0.0}}] -> w602
        tunnel: w596 -> [w624 _]
        tunnel: [w629 _] -> w595
        tunnel: w594 -> [w626 _]
        tunnel: [w623 _] -> w593
        frame No Error {
          n260 = Unbundle By Name(w658) -> ("Reference System"=w657:T36, "Measurement System"=w656:T36)
          n261 = Unbundle By Name(w659) -> ("Clamp Points.Pixels"=w662:T77)
          n262 = Unbundle By Name(w662) -> ("Start.X"=w655:dbl, "Start.Y"=w654:dbl, "End.X"=w653:dbl, "End.Y"=w652:dbl)
          n263 = Add(x=w655, y=w661) -> (x+y=w651:dbl)
          n264 = Add(x=w654, y=w660) -> (x+y=w650:dbl)
          n265 = Add(x=w653, y=w661) -> (x+y=w649:dbl)
          n266 = Add(x=w652, y=w660) -> (x+y=w648:dbl)
          n267 = Bundle(w651, w650) -> (w628:cluster{dbl, dbl})  [unwired: 1 in]
          n268 = Bundle(w649, w648) -> (w627:cluster{dbl, dbl})  [unwired: 1 in]
          n269 = call "IMAQ Convert Point to ROI"("Point"=w628) -> ("ROI Descriptor"=w647:T12)  [unwired: 8 in, 1 out]
          n270 = call "IMAQ Convert Point to ROI"("Point"=w627) -> ("ROI Descriptor"=w646:T12)  [unwired: 8 in, 1 out]
          n271 = call "IMAQ TransformROI"("New Reference"=w656, "Base Reference"=w657, "ROI Descriptor"=w647) -> ("ROI Descriptor out"=w645:T12)  [unwired: 7 in, 1 out]
          n272 = call "IMAQ TransformROI"("New Reference"=w656, "Base Reference"=w657, "ROI Descriptor"=w646) -> ("ROI Descriptor out"=w644:T12)  [unwired: 7 in, 1 out]
          n273 = Build Array(w628, w627) -> (w625:cluster{dbl, dbl}[])
          n274 = call "IMAQ Convert ROI to Point"("ROI Descriptor"=w645) -> ("Point"=w642:T15)  [unwired: 8 in, 1 out]
          n275 = call "IMAQ Convert ROI to Point"("ROI Descriptor"=w644) -> ("Point"=w641:T15)  [unwired: 8 in, 1 out]
          n276 = Build Array(w642, w641) -> (w630:T15[])
          n277 = call "IMAQ Convert Pixel to Real World"("Array of Pixel Coordinates"=w630, "Calibrated Image"=w643) -> ("error out"=w631:errorcluster, "Array of Real World Coordinates"=w637:cluster{"X":sgl, "Y":sgl}[])  [unwired: 4 in, 4 out]
          n278 = case shown="True" w626 {
            tunnel: w624 -> [w670 w677]
            tunnel: w630 -> [_ w678]
            tunnel: [w669 w676] -> w629
            tunnel: w625 -> [w668 _]
            frame False {
              n279 = for {
                tunnel: w668 -> [w675] mode=indexing
                tunnel: w670 -> [w674]
                tunnel: [w671] -> w669 mode=indexing
                n280 = Unbundle(w675) -> (w673:dbl, w672:dbl)
                n281 = Bundle(w674, w673, w672) -> (w671:cluster{string, dbl, dbl})  [unwired: 1 in]
              }
            }
            frame True {
              n282 = for {
                tunnel: w678 -> [w683] mode=indexing
                tunnel: w677 -> [w682]
                tunnel: [w679] -> w676 mode=indexing
                n283 = Unbundle(w683) -> ("X"=w681:sgl, "Y"=w680:sgl)
                n284 = Bundle(w682, "X"=w681, "Y"=w680) -> (w679:cluster{string, "X":sgl, "Y":sgl})  [unwired: 1 in]
              }
            }
          }
          n285 = call <vilib>:"Clear Errors.vi"("error in (no error)"=w631) -> ()  [unwired: 5 in, 2 out]
          n286 = Bundle("Point"=w642, "Point"=w641) -> (w640:cluster{"Point":T15, "Point":T15})  [unwired: 1 in]
          n287 = call "IMAQ Point Distances"("Points"=w637) -> ("Distances"=w639:sgl[])  [unwired: 4 in, 1 out]
          n288 = Index Array(array=w637, index #1=0 ("index"), index #2=1 ("index")) -> (element #1=w634:cluster{"X":sgl, "Y":sgl}, element #2=w633:cluster{"X":sgl, "Y":sgl})
          n289 = for {
            tunnel: w625 -> [w667] mode=indexing
            tunnel: w624 -> [w666]
            tunnel: [w663] -> w623 mode=indexing
            n290 = Unbundle(w667) -> (w665:dbl, w664:dbl)
            n291 = Bundle(w666, w665, w664) -> (w663:cluster{string, dbl, dbl})  [unwired: 1 in]
          }
          n292 = Index Array(array=w639) -> (element=w638:sgl)  [unwired: 1 in]
          n293 = Bundle(w634, w633) -> (w632:T22)  [unwired: 1 in]
        }
        frame Error {
        }
      }
      n294 = Bundle By Name(cluster=w605, "Clamp Points.Pixels"=w604, "Clamp Results.Distance (Real World)"=w603, "Clamp Points.Real World"=w602) -> (w601:T76)
      n295 = To Variant(anything=w601) -> (Variant=w610:variant)
    }
    frame 7 {
      w702 = "_" ("string")
      w720 = T78 {"Selected Particle"=0, "Connectivity 4/8 (8)"=TRUE, "MaxParticle"=0}  # Analysis_Particle_Parameter
      n296 = Variant To Data(type=w720, Variant=w721) -> (data=w719:T78)  [unwired: 1 in, 1 out]
      n297 = Unbundle By Name(w719) -> ("Selected Particle"=w717:i32, "Connectivity 4/8 (8)"=w705:bool, "MaxParticle"=w694:i32)
      n298 = Concatenate Strings(w700, w702, w701, w702, "Particle" ("string")) -> (w699:string)
      n299 = call "Particle_Main Function.vi"("ForCalCalculaton In"=w706, "MAXParticle"=w694, "error in (no error)"=w713, "Connectivity 4/8 (8)"=w705, "Selected Particle"=w717, "Refnum in"=w718) -> ("error out"=w712:errorcluster, "Particle Reports (Real-World)"=w708:T79, "Particle Report"=w696:T79, "Refnum out"=w710:T2, "SearchSize"=w695:i32)  [unwired: 1 in]
      n300 = Max & Min(x=w694, y=w695) -> (min(x,y)=w693:i32)  [unwired: 1 out]
      n301 = for {
        N: w693 -> [_]
        tunnel: w716 -> [w738]
        tunnel: w715 -> [w737]
        tunnel: w712 -> [w736]
        tunnel: w711 -> [w735]
        tunnel: w696 -> [w726]
        tunnel: [w732] -> w689 mode=indexing
        tunnel: w708 -> [w724]
        tunnel: [w731] -> w707 mode=indexing
        tunnel: w704 -> [w730]
        tunnel: w699 -> [w729]
        tunnel: [w728] -> w698 mode=indexing
        tunnel: [w727] -> w697 mode=indexing
        i -> [w722]
        # "Pixel"
        # "Real World"
        n302 = Index Array(array=w724, index=w722) -> (element=w723:T23)
        n303 = Index Array(array=w726, index=w722) -> (element=w725:T23)
        n304 = case shown="No Error" w736 {
          tunnel: w738 -> [w763 _]
          tunnel: w737 -> [w762 _]
          tunnel: w725 -> [w767 _]
          tunnel: w735 -> [w777 _]
          tunnel: [w769 T24 {"Left"=0.0, "Top"=0.0, "Right"=0.0, "Bottom"=0.0} ("Bounding Rect")] -> w734
          tunnel: [w768 T15 {"X"=0.0, "Y"=0.0} ("Point")] -> w733
          tunnel: [w746 T23 {"Area"=0.0, "Number of Holes"=0.0, "Bounding Rect"={"Left"=0.0, "Top"=0.0, "Right"=0.0, "Bottom"=0.0}, "Center of Mass"={"X"=0.0, "Y"=0.0}, "Orientation"=0.0, "Dimensions"={"Width"=0.0, "Height"=0.0}} ("Particle Report")] -> w731
          tunnel: w723 -> [w746 _]
          tunnel: w730 -> [w747 _]
          tunnel: w722 -> [w753 _]
          tunnel: w729 -> [w751 _]
          tunnel: [w748 _] -> w728
          tunnel: [w740 _] -> w727
          frame No Error {
            n305 = Unbundle By Name(w767) -> ("Bounding Rect"=w788:T24, "Center of Mass"=w764:cluster{"X":dbl, "Y":dbl})
            n306 = Unbundle By Name(w777) -> ("Reference System"=w772:T36, "Measurement System"=w771:T36)
            n307 = Unbundle By Name(w746) -> ("Center of Mass.X"=w745:dbl, "Center of Mass.Y"=w744:dbl)
            n308 = Increment(x=w753) -> (x+1=w754:i32)
            n309 = Unbundle By Name(w788) -> ("Left"=w757:dbl, "Top"=w756:dbl, "Right"=w758:dbl, "Bottom"=w755:dbl)
            n310 = Unbundle By Name(w764) -> ("X"=w743:dbl, "Y"=w742:dbl)
            n311 = Number To Decimal String(number=w754) -> (decimal integer string=w752:string)  [unwired: 1 in]
            n312 = Add(x=w742, y=w762) -> (x+y=w760:dbl)
            n313 = Concatenate Strings(w751, w752) -> (w741:string)
            n314 = Add(x=w743, y=w763) -> (x+y=w761:dbl)
            n315 = Add(x=w757, y=w763) -> (x+y=w786:dbl)
            n316 = Add(x=w756, y=w762) -> (x+y=w787:dbl)
            n317 = Add(x=w758, y=w763) -> (x+y=w784:dbl)
            n318 = Add(x=w755, y=w762) -> (x+y=w783:dbl)
            n319 = Bundle(w761, w760) -> (w759:cluster{dbl, dbl})  [unwired: 1 in]
            n320 = Bundle(w784, w783) -> (w782:cluster{dbl, dbl})  [unwired: 1 in]
            n321 = Bundle(w786, w787) -> (w785:cluster{dbl, dbl})  [unwired: 1 in]
            n322 = call "IMAQ Convert Point to ROI"("Point"=w782) -> ("ROI Descriptor"=w780:T12)  [unwired: 8 in, 1 out]
            n323 = call "IMAQ Convert Point to ROI"("Point"=w785) -> ("ROI Descriptor"=w781:T12)  [unwired: 8 in, 1 out]
            n324 = call "IMAQ Convert Point to ROI"("Point"=w759) -> ("ROI Descriptor"=w773:T12)  [unwired: 8 in, 1 out]
            n325 = call "IMAQ TransformROI"("New Reference"=w771, "Base Reference"=w772, "ROI Descriptor"=w773) -> ("ROI Descriptor out"=w770:T12)  [unwired: 7 in, 1 out]
            n326 = call "IMAQ TransformROI"("New Reference"=w771, "Base Reference"=w772, "ROI Descriptor"=w780) -> ("ROI Descriptor out"=w778:T12)  [unwired: 7 in, 1 out]
            n327 = call "IMAQ TransformROI"("New Reference"=w771, "Base Reference"=w772, "ROI Descriptor"=w781) -> ("ROI Descriptor out"=w779:T12)  [unwired: 7 in, 1 out]
            n328 = case shown="False" w747 {
              tunnel: [w790 w792] -> w750
              tunnel: w743 -> [w790 _]
              tunnel: [w789 w791] -> w749
              tunnel: w742 -> [w789 _]
              tunnel: w745 -> [_ w792]
              tunnel: w744 -> [_ w791]
              frame False {
              }
              frame True {
              }
            }
            n329 = call "IMAQ Convert ROI to Point"("ROI Descriptor"=w770) -> ("Point"=w768:T15)  [unwired: 8 in, 1 out]
            n330 = call "IMAQ Convert ROI to Point"("ROI Descriptor"=w779) -> ("Point"=w766:T15)  [unwired: 8 in, 1 out]
            n331 = call "IMAQ Convert ROI to Point"("ROI Descriptor"=w778) -> ("Point"=w765:T15)  [unwired: 8 in, 1 out]
            n332 = Bundle(w741, "X"=w743, "Y"=w742) -> (w740:cluster{string, "X":dbl, "Y":dbl})  [unwired: 1 in]
            n333 = Unbundle(w766) -> ("X"=w776:sgl, "Y"=w775:sgl)
            n334 = Unbundle(w765) -> ("X"=w739:sgl, "Y"=w774:sgl)
            n335 = Bundle By Name(cluster=w788, "Left"=w776, "Top"=w775, "Right"=w739, "Bottom"=w774) -> (w769:T24)
            n336 = Bundle(w741, "X"=w750, "Y"=w749) -> (w748:cluster{string, "X":dbl, "Y":dbl})  [unwired: 1 in]
          }
          frame Error {
          }
        }
        n337 = Bundle By Name(cluster=w725, "Bounding Rect"=w734, "Center of Mass"=w733) -> (w732:T23)
      }
      n338 = Subtract(x=w694, y=w693) -> (x-y=w692:i32)
      n339 = Initialize Array(T23 {"Area"=0.0, "Number of Holes"=0.0, "Bounding Rect"={"Left"=0.0, "Top"=0.0, "Right"=0.0, "Bottom"=0.0}, "Center of Mass"={"X"=0.0, "Y"=0.0}, "Orientation"=0.0, "Dimensions"={"Width"=0.0, "Height"=0.0}} ("Particle Report"), w692) -> (w687:T79)
      n340 = Build Array (concatenate)(w689, w687) -> (w690:T79)
      n341 = Build Array (concatenate)(w707, w687) -> (w688:T79)
      n342 = Bundle(w690, w688) -> (w709:T80)  [unwired: 1 in]
      n343 = To Variant(anything=w709) -> (Variant=w714:variant)
    }
    frame 8 {
      w805 = T81 {"Interval Range"={"Minimum"=0.0, "Maximum"=0.0}, "ROI Out"={"Global Rectangle"=[], "Contours"=[]}, "Number of Classes"=256}  # Analysis_Histogram_Parameter
      n344 = Variant To Data(type=w805, Variant=w808) -> (data=w806:T81)  [unwired: 1 in, 1 out]
      n345 = Unbundle By Name(w806) -> ("Number of Classes"=w802:i32, "Interval Range"=w803:cluster{"Minimum":sgl, "Maximum":sgl}, "ROI Out"=w796:T41)
      n346 = call "Histogram_Main Function.vi"("ROI Descriptor"=w796, "Number of Classes"=w802, "error in (no error)"=w798, "Interval Range"=w803, "Refnum in"=w804) -> ("error out"=w797:errorcluster, "Histogram Report"=w800:T82, "Refnum out"=w801:T2)  [unwired: 4 in]
      n347 = Bundle("Histogram Report"=w800, "ROI Out"=w796) -> (w799:T83)  [unwired: 1 in]
      n348 = To Variant(anything=w799) -> (Variant=w807:variant)
    }
    frame 9 {
      (unwired) cluster{string, "X":sgl, "Y":sgl}[] [] ("appended array")
      w829 = T84 {"ROI Descriptor"={"Global Rectangle"=[], "Contours"=[]}, "Number of Matches Requested"=1, "Edge Info Size"=0, "Options"={"Search Direction"=0, "Edge Options"={"Edge Polarity"=0, "Kernel Size"=3, "Width"=3, "Minimum Edge Strength"=10.0, "Interpolation Type"=enum."Bilinear Fixed", "Data Processing Method"=enum."Average"}, "Show Search Area"=FALSE, "Show Search Lines"=FALSE, "Show Edges Found"=FALSE, "Show Result"=TRUE, "Search Area Color"=65280, "Search Lines Color"=255, "Edge Locations Color"=16776960, "Result Color"=16711680, "Overlay Group Name"=""}, "Line Fit Options"={"Number of Lines"=1, "Type"=enum."First Edge Rake", "Min. Score"=10.0, "Max. Score"=1000.0, "Orientation"=0.0, "Angle Range"=45.0, "Angle Tolerance"=1.0, "Step Size"=7, "Min. SNR (db)"=0.0, "Min. Points (%)"=25.0, "Hough Iterations"=5}}  # Analysis_Find Straight Edge_Parameter
      w832 = "_" ("string")
      n349 = Variant To Data(type=w829, Variant=w830) -> (data=w828:T84)  [unwired: 1 in, 1 out]
      n350 = Concatenate Strings(w831, w832, w809, w832, "Edge" ("string")) -> (w822:string)
      n351 = Unbundle By Name(w828) -> ("Number of Matches Requested"=w810:i32, "Options"=w827:T89, "Line Fit Options"=w826:T87, "ROI Descriptor"=w818:T41)
      n352 = call "Find Straight Edge_Main Function.vi"("Refnum in"=w817, "Number of Matches Requested"=w810, "Options"=w827, "Line Fit Options"=w826, "error in (no error)"=w816, "ROI"=w818) -> ("Refnum out"=w813:T2, "Straight Edges"=w825:T90, "error out"=w815:errorcluster)  [unwired: 7 in]
      n353 = case shown="No Error" w815 {
        tunnel: w825 -> [w836 _]
        tunnel: w824 -> [w845 _]
        tunnel: w823 -> [w844 _]
        tunnel: w822 -> [w843 _]
        tunnel: [w842 w929] -> w821
        tunnel: [w841 w931] -> w819
        tunnel: w814 -> [w840 _]
        tunnel: w813 -> [w839 _]
        tunnel: w812 -> [w838 _]
        tunnel: [w837 w924] -> w811
        tunnel: w810 -> [w835 w927]
        frame No Error {
          n354 = Empty Array?(array=w836) -> (empty?=w834:bool)
          n355 = for {
            N: w835 -> [_]
            tunnel: w836 -> [w905]
            tunnel: w845 -> [w898]
            tunnel: w844 -> [w897]
            tunnel: [w904] -> w841 mode=indexing
            tunnel: w843 -> [w899]
            tunnel: [w891] -> w842 mode=concatenating
            tunnel: w840 -> [w890]
            tunnel: w839 -> [w877]
            tunnel: w838 -> [w871]
            tunnel: [w858] -> w837 mode=concatenating
            tunnel: w834 -> [w847]
            i -> [w856]
            w846 = T15 {"X"=-1.0, "Y"=-1.0} ("t")
            n356 = Increment(x=w856) -> (x+1=w901:i32)
            n357 = Index Array(array=w905, index=w856) -> (element=w857:T25)
            n358 = Unbundle By Name(w857) -> ("Point1 (Pixels).X"=w907:sgl, "Point1 (Pixels).Y"=w906:sgl, "Point2 (Pixels).X"=w903:sgl, "Point2 (Pixels).Y"=w902:sgl)
            n359 = Unbundle By Name(w890) -> ("Reference System"=w881:T36, "Measurement System"=w880:T36)
            n360 = Number To Decimal String(number=w901) -> (decimal integer string=w900:string)  [unwired: 1 in]
            n361 = Concatenate Strings(w899, w900) -> (w895:string)
            n362 = Concatenate Strings(w895, ".P1" ("string")) -> (w866:string)
            n363 = Concatenate Strings(w895, ".P2" ("string")) -> (w865:string)
            n364 = Add(x=w907, y=w898) -> (x+y=w889:sgl)
            n365 = Add(x=w906, y=w897) -> (x+y=w888:sgl)
            n366 = Add(x=w903, y=w898) -> (x+y=w887:sgl)
            n367 = Add(x=w902, y=w897) -> (x+y=w886:sgl)
            n368 = Bundle(w889, w888) -> (w885:cluster{sgl, sgl})  [unwired: 1 in]
            n369 = Bundle(w887, w886) -> (w884:cluster{sgl, sgl})  [unwired: 1 in]
            n370 = call "IMAQ Convert Point to ROI"("Point"=w884) -> ("ROI Descriptor"=w882:T12)  [unwired: 8 in, 1 out]
            n371 = call "IMAQ Convert Point to ROI"("Point"=w885) -> ("ROI Descriptor"=w883:T12)  [unwired: 8 in, 1 out]
            n372 = call "IMAQ TransformROI"("New Reference"=w880, "Base Reference"=w881, "ROI Descriptor"=w883) -> ("ROI Descriptor out"=w879:T12)  [unwired: 7 in, 1 out]
            n373 = call "IMAQ TransformROI"("New Reference"=w880, "Base Reference"=w881, "ROI Descriptor"=w882) -> ("ROI Descriptor out"=w878:T12)  [unwired: 7 in, 1 out]
            n374 = call "IMAQ Convert ROI to Point"("ROI Descriptor"=w879) -> ("Point"=w855:T15)  [unwired: 8 in, 1 out]
            n375 = call "IMAQ Convert ROI to Point"("ROI Descriptor"=w878) -> ("Point"=w853:T15)  [unwired: 8 in, 1 out]
            n376 = Build Array(w855, w853) -> (w876:T15[])
            n377 = call "IMAQ Convert Pixel to Real World"("Array of Pixel Coordinates"=w876, "Calibrated Image"=w877) -> ("error out"=w875:errorcluster, "Array of Real World Coordinates"=w874:cluster{"X":sgl, "Y":sgl}[])  [unwired: 4 in, 4 out]
            n378 = call <vilib>:"Clear Errors.vi"("error in (no error)"=w875) -> ()  [unwired: 5 in, 2 out]
            n379 = Select(t=w846, s=w847, f=w855) -> (s? t:f=w854:T15)
            n380 = Select(t=w846, s=w847, f=w853) -> (s? t:f=w852:T15)
            n381 = Index Array(array=w874, index #1=0 ("index"), index #2=1 ("index")) -> (element #1=w851:cluster{"X":sgl, "Y":sgl}, element #2=w849:cluster{"X":sgl, "Y":sgl})
            n382 = Select(t=w846, s=w847, f=w851) -> (s? t:f=w850:T15)
            n383 = Select(t=w846, s=w847, f=w849) -> (s? t:f=w848:T15)
            n384 = Unbundle(w854) -> ("X"=w864:sgl, "Y"=w863:sgl)
            n385 = Unbundle(w852) -> ("X"=w862:sgl, "Y"=w861:sgl)
            n386 = Unbundle(w850) -> ("X"=w870:sgl, "Y"=w869:sgl)
            n387 = Unbundle(w848) -> ("X"=w868:sgl, "Y"=w867:sgl)
            n388 = case shown="True" w871 {
              tunnel: w866 -> [w915 w923]
              tunnel: w865 -> [w914 w922]
              tunnel: [w913 w916] -> w894
              tunnel: [w912 w917] -> w893
              tunnel: w864 -> [w911 _]
              tunnel: w863 -> [w910 _]
              tunnel: w862 -> [w909 _]
              tunnel: w861 -> [w908 _]
              tunnel: w870 -> [_ w921]
              tunnel: w869 -> [_ w920]
              tunnel: w868 -> [_ w919]
              tunnel: w867 -> [_ w918]
              frame False {
                n389 = Bundle(w915, "X"=w911, "Y"=w910) -> (w913:cluster{string, "X":sgl, "Y":sgl})  [unwired: 1 in]
                n390 = Bundle(w914, "X"=w909, "Y"=w908) -> (w912:cluster{string, "X":sgl, "Y":sgl})  [unwired: 1 in]
              }
              frame True {
                n391 = Bundle(w922, "X"=w919, "Y"=w918) -> (w917:cluster{string, "X":sgl, "Y":sgl})  [unwired: 1 in]
                n392 = Bundle(w923, "X"=w921, "Y"=w920) -> (w916:cluster{string, "X":sgl, "Y":sgl})  [unwired: 1 in]
              }
            }
            n393 = Bundle(w866, "X"=w864, "Y"=w863) -> (w860:cluster{string, "X":sgl, "Y":sgl})  [unwired: 1 in]
            n394 = Bundle(w865, "X"=w862, "Y"=w861) -> (w859:cluster{string, "X":sgl, "Y":sgl})  [unwired: 1 in]
            n395 = Build Array(w860, w859) -> (w858:cluster{string, "X":sgl, "Y":sgl}[])
            n396 = Bundle By Name(cluster=w857, "Point1 (Pixels).X"=w864, "Point1 (Pixels).Y"=w863, "Point2 (Pixels).X"=w862, "Point2 (Pixels).Y"=w861, "Point1 (Real-World)"=w850, "Point2 (Real-World)"=w848) -> (w904:T25)
            n397 = Build Array(w894, w893) -> (w891:cluster{string, "X":sgl, "Y":sgl}[])
          }
        }
        frame Error {
          (unwired) T90 []
          (unwired) cluster{string, sgl, sgl}[] []
          n398 = Multiply(x=w927, y=2) -> (x*y=w925:i32)
          n399 = Initialize Array(T25 {"Point1 (Pixels)"={"X"=0.0, "Y"=0.0}, "Point2 (Pixels)"={"X"=0.0, "Y"=0.0}, "Point1 (Real-World)"={"X"=0.0, "Y"=0.0}, "Point2 (Real-World)"={"X"=0.0, "Y"=0.0}, "Angle (Pixel)"=0.0, "Angle (Real-World)"=0.0, "Score"=0.0, "Straightness"=0.0, "Average SNR (db)"=0.0, "Calibration Valid"=FALSE} ("Cluster"), w927) -> (w931:T90)
          n400 = Initialize Array(cluster{string, sgl, sgl} {"", 0.0, 0.0}, w927) -> (w929:cluster{string, sgl, sgl}[])
          n401 = Initialize Array(cluster{string, "X":sgl, "Y":sgl} {"", "X"=0.0, "Y"=0.0}, w925) -> (w924:cluster{string, "X":sgl, "Y":sgl}[])
        }
      }
      n402 = To Variant(anything=w819) -> (Variant=w820:variant)
    }
    frame 10 {
      w953 = "_" ("string")
      w979 = T91 {"ROI Descriptor"={"Global Rectangle"=[], "Contours"=[]}, "Options"={"Search  Direction"=0, "Edge Options"={"Edge Polarity"=0, "Kernel Size"=3, "Width"=3, "Minimum Edge Strength"=10.0, "Interpolation Type"=enum."Bilinear Fixed", "Data Processing Method"=enum."Average"}, "Show Search Area"=FALSE, "Show Search Lines"=FALSE, "Show Edges Found"=FALSE, "Show Result"=TRUE, "Search Area Color"=65280, "Search Lines Color"=255, "Edge Locations Color"=16776960, "Result Color"=16711680, "Overlay Group Name"=""}, "Circle Fit Options"={"Process"=enum."Get First Edge", "Step Size"=3.0, "Max Pixel Radius"=3}}  # Analysis_Circle_Parameter
      n403 = Variant To Data(type=w979, Variant=w981) -> (data=w980:T91)  [unwired: 1 in, 1 out]
      n404 = Unbundle By Name(w980) -> ("Options"=w976:T92, "ROI Descriptor"=w974:T41, "Circle Fit Options"=w977:T93)
      n405 = Unbundle By Name(w972) -> ("Reference System"=w960:T36, "Measurement System"=w959:T36)
      n406 = call "Circle_Main Function.vi"("Refnum in"=w978, "Circle Fit Options"=w977, "ROI"=w974, "Options"=w976, "error in (no error)"=w975) -> ("Refnum out"=w937:T2, "Fitted Circle"=w955:T94)  [unwired: 12 in, 1 out]
      n407 = Concatenate Strings(w951, w953, w950, w953, "Circle" ("string")) -> (w943:string)
      n408 = Unbundle By Name(w955) -> ("Center (Pixels)"=w967:cluster{"X":sgl, "Y":sgl}, "Radius (Pixels)"=w968:dbl)
      n409 = Unbundle By Name(w967) -> ("X"=w965:sgl, "Y"=w966:sgl)
      n410 = Add(x=w964, y=w965) -> (x+y=w948:sgl)
      n411 = Add(x=w963, y=w966) -> (x+y=w947:sgl)
      n412 = Bundle By Name(cluster=T26 {"Center X"=0, "Center Y"=0, "Inner Radius"=0, "Outer Radius"=0, "Start Angle"=0.0, "End Angle"=0.0} ("Annulus"), "Center X"=w948, "Center Y"=w947, "Start Angle"=0.0, "End Angle"=360 ("Outer Radius"), "Inner Radius"=w968, "Outer Radius"=w968) -> (w957:T26)
      n413 = Bundle(w948, w947) -> (w935:cluster{sgl, sgl})  [unwired: 1 in]
      n414 = call "IMAQ Convert Annulus to ROI"("Annulus"=w957) -> ("ROI Descriptor"=w962:T12)  [unwired: 8 in, 1 out]
      n415 = call "IMAQ Convert Point to ROI"("Point"=w935) -> ("ROI Descriptor"=w961:T12)  [unwired: 8 in, 1 out]
      n416 = call "IMAQ TransformROI"("New Reference"=w959, "Base Reference"=w960, "ROI Descriptor"=w962) -> ("ROI Descriptor out"=w958:T12)  [unwired: 7 in, 1 out]
      n417 = call "IMAQ TransformROI"("New Reference"=w959, "Base Reference"=w960, "ROI Descriptor"=w961) -> ("ROI Descriptor out"=w936:T12)  [unwired: 7 in, 1 out]
      n418 = call "IMAQ Convert ROI to Point"("ROI Descriptor"=w936) -> ("Point"=w933:T15)  [unwired: 8 in, 1 out]
      n419 = call "IMAQ Convert Pixel to Real World"("Pixel Coordinates"=w933, "Calibrated Image"=w937) -> ("error out"=w938:errorcluster, "Real World Coordinates"=w934:cluster{"X":sgl, "Y":sgl})  [unwired: 4 in, 4 out]
      n420 = Bundle By Name(cluster=w955, "Center (Pixels)"=w933, "Center (Real-World)"=w934) -> (w954:T94)
      n421 = Bundle("ROI Descriptor out"=w958, "ROI Descriptor out"=w936, "Fitted Circle"=w954) -> (w956:T95)  [unwired: 1 in]
      n422 = To Variant(anything=w956) -> (Variant=w973:variant)
      n423 = call <vilib>:"Clear Errors.vi"("error in (no error)"=w938) -> ()  [unwired: 5 in, 2 out]
      n424 = Unbundle(w933) -> ("X"=w945:sgl, "Y"=w944:sgl)
      n425 = Bundle(cluster=cluster{string, "X":dbl, "Y":dbl} {"", "X"=0.0, "Y"=0.0}, w943, "X"=w945, "Y"=w944) -> (w940:cluster{string, "X":dbl, "Y":dbl})
      n426 = Bundle(cluster=cluster{string, "X":dbl, "Y":dbl} {"", "X"=0.0, "Y"=0.0}, w943, "X"=w948, "Y"=w947) -> (w942:cluster{string, "X":dbl, "Y":dbl})
      n427 = Build Array(w940) -> (w939:cluster{string, "X":dbl, "Y":dbl}[])
      n428 = Build Array(w942) -> (w941:cluster{string, "X":dbl, "Y":dbl}[])
    }
    frame 11 {
      (unwired) T96 {"Pixel"=[{"Position"={"X"=523.69354, "Y"=1003.37823}, "Angle"=197.96374516862053, "Major Radius"=397.8460760350613, "Minor Radius"=117.08356439471159, "Score"=989.1618691264235}], "Ellipses (Calibrated)"=[{"Position"={"X"=523.69354, "Y"=1003.37823}, "Orientation"=197.96374516862053, "Major Radius"=397.8460760350613, "Minor Radius"=117.08356439471159, "Score"=989.1618691264235}]}  # Ellipses
      w1002 = "_" ("string")
      n429 = Variant To Data(type=T27 {"Enum_ShapeType"=enum."Circles", "MaxParticle"=1, "Descriptor"={"Set 1"=100.0, "Set 2"=10.0, "Set 3"=200.0, "Set 4"=10.0}, "Match Options"={"Rotation"=TRUE, "Scale"=FALSE, "Occlusion"=FALSE, "Range Settings"=[{"Match Constraints"=0, "Min"=0.0, "Max"=360.0}]}, "Curve Parameters"={"Extraction Mode"=0, "Edge Threshold"=75, "Edge Filter Size"=1, "Min Length"=25, "Row Search Step Size"=15, "Col Search Step Size"=15, "Max Endpoint Gap"=10, "Closed"=FALSE, "Subpixel"=FALSE}, " score"=500.0} ("SetParameter"), Variant=w983) -> (data=w982:T27)  [unwired: 1 in, 1 out]
      n430 = Concatenate Strings(w1000, w1002, w999, w1002, "Shape" ("string")) -> (w993:string)
      n431 = call "ShapeDectect.vi"("error in (no error)"=w986, "SetParameter"=w982, "Image In"=w984) -> ("DectectItem"=w987:i32, "ResultOut"=w996:variant)  [unwired: 5 in, 2 out]
      n432 = Unbundle By Name(w982) -> ("Enum_ShapeType"=w997:T97)
      n433 = Unbundle By Name(w1003) -> ("Reference System"=w989:T36, "Measurement System"=w991:T36)
      n434 = case shown="\"Ellipses\"" w997 {
        selector: w997 -> [w1007 w1068 w1116 w1202]
        tunnel: w996 -> [w1020 w1080 w1132 w1218]
        tunnel: w995 -> [w1017 w1077 w1129 w1215]
        tunnel: w994 -> [w1016 w1076 w1128 w1214]
        tunnel: w984 -> [w1014 w1074 w1126 w1212]
        tunnel: w993 -> [w1008 w1069 w1119 w1206]
        tunnel: [w1013 w1073 w1125 w1211] -> w992
        tunnel: [w1012 w1072 w1124 w1210] -> w990
        tunnel: w989 -> [w1011 w1064 w1123 w1209]
        tunnel: w991 -> [w1010 w1063 w1122 w1208]
        tunnel: [w1009 w1071 w1121 w1207] -> w988
        tunnel: w987 -> [w1006 w1067 w1115 w1198]
        tunnel: w985 -> [_ _ _ w1199]
        frame "Circles", Default {
          w1021 = T98 {"Circles"=[{"Position"={"X"=1609.8834, "Y"=1004.1779}, "Radius"=276.62862303147017, "Score"=988.8745123015594}], "Circles (Calibrated)"=[{"Position"={"X"=1609.8834, "Y"=1004.1779}, "Radius"=276.62862303147017, "Score"=988.8745123015594}]}  # Circles
          n435 = Variant To Data(type=w1021, Variant=w1020) -> (data=w1019:T98)  [unwired: 1 in, 1 out]
          n436 = Unbundle(w1019) -> ("Circles"=w1018:T99, "Circles (Calibrated)"=w1015:T99)
          n437 = for {
            tunnel: w1018 -> [w1058] mode=indexing
            tunnel: w1017 -> [w1060]
            tunnel: w1016 -> [w1059]
            tunnel: w1015 -> [w1056] mode=indexing
            tunnel: w1014 -> [w1057]
            tunnel: [w1054] -> w1013 mode=indexing
            tunnel: [w1049] -> w1012 mode=indexing
            tunnel: w1011 -> [w1024]
            tunnel: w1010 -> [w1023]
            tunnel: [w1037] -> w1005 mode=indexing
            tunnel: w1008 -> [w1035]
            i -> [w1034]
            n438 = Increment(x=w1034) -> (x+1=w1033:i32)
            n439 = Unbundle By Name(w1058) -> ("Position.X"=w1062:sgl, "Position.Y"=w1061:sgl, "Radius"=w1043:dbl)  [unwired: 1 out]
            n440 = Number To Decimal String(number=w1033) -> (decimal integer string=w1032:string)  [unwired: 1 in]
            n441 = Concatenate Strings(w1035, " Circles" ("string"), w1032) -> (w1031:string)
            n442 = Add(x=w1060, y=w1062) -> (x+y=w1048:sgl)
            n443 = Add(x=w1059, y=w1061) -> (x+y=w1047:sgl)
            n444 = Bundle(w1048, w1047) -> (w1025:cluster{sgl, sgl})  [unwired: 1 in]
            n445 = Bundle(cluster=cluster{string, "X":dbl, "Y":dbl} {"", "X"=0.0, "Y"=0.0}, w1031, "X"=w1048, "Y"=w1047) -> (w1054:cluster{string, "X":dbl, "Y":dbl})
            n446 = Bundle(cluster=T26 {"Center X"=0, "Center Y"=0, "Inner Radius"=0, "Outer Radius"=0, "Start Angle"=0.0, "End Angle"=0.0} ("Annulus"), "Center X"=w1048, "Center Y"=w1047, "Inner Radius"=w1043, "Outer Radius"=w1043, "Start Angle"=0.0, "End Angle"=360.0) -> (w1044:T26)
            n447 = call "IMAQ Convert Annulus to ROI"("Annulus"=w1044) -> ("ROI Descriptor"=w1046:T12)  [unwired: 8 in, 1 out]
            n448 = call "IMAQ Convert Point to ROI"("Point"=w1025) -> ("error out"=w1026:errorcluster, "ROI Descriptor"=w1029:T12)  [unwired: 8 in]
            n449 = call "IMAQ TransformROI"("error in (no error)"=w1026, "New Reference"=w1023, "Base Reference"=w1024, "ROI Descriptor"=w1029) -> ("error out"=w1027:errorcluster, "ROI Descriptor out"=w1028:T12)  [unwired: 6 in]
            n450 = call "IMAQ TransformROI"("New Reference"=w1023, "Base Reference"=w1024, "ROI Descriptor"=w1046) -> ("ROI Descriptor out"=w1039:T12)  [unwired: 7 in, 1 out]
            n451 = call "IMAQ Convert ROI to Point"("error in (no error)"=w1027, "ROI Descriptor"=w1028) -> ("Point"=w1022:T15)  [unwired: 7 in, 1 out]
            n452 = call "IMAQ Convert Pixel to Real World"("Pixel Coordinates"=w1022, "Calibrated Image"=w1057) -> ("error out"=w1030:errorcluster, "Real World Coordinates"=w1053:cluster{"X":sgl, "Y":sgl})  [unwired: 4 in, 4 out]
            n453 = Bundle By Name(cluster=w1058, "Position"=w1022) -> (w1040:T100)
            n454 = Bundle By Name(cluster=w1056, "Position"=w1053) -> (w1038:T100)
            n455 = call <vilib>:"Clear Errors.vi"("error in (no error)"=w1030) -> ()  [unwired: 5 in, 2 out]
            n456 = Unbundle(w1053) -> ("X"=w1051:sgl, "Y"=w1050:sgl)
            n457 = Bundle(cluster=cluster{string, "X":dbl, "Y":dbl} {"", "X"=0.0, "Y"=0.0}, w1031, "X"=w1051, "Y"=w1050) -> (w1049:cluster{string, "X":dbl, "Y":dbl})
            n458 = Bundle("ROI Descriptor out"=w1039, "Circle Descriptor"=w1040, "Circle Descriptor"=w1038) -> (w1037:T101)  [unwired: 1 in]
          }
          n459 = Bundle("Enum_ShapeType"=w1007, "DectectItem"=w1006, w1005) -> (w1004:T102)  [unwired: 1 in]
          n460 = To Variant(anything=w1004) -> (Variant=w1009:variant)
        }
        frame "Ellipses" {
          w1070 = T96 {"Pixel"=[{"Position"={"X"=523.69354, "Y"=1003.37823}, "Angle"=197.96374516862053, "Major Radius"=397.8460760350613, "Minor Radius"=117.08356439471159, "Score"=989.1618691264235}], "Ellipses (Calibrated)"=[{"Position"={"X"=523.69354, "Y"=1003.37823}, "Orientation"=197.96374516862053, "Major Radius"=397.8460760350613, "Minor Radius"=117.08356439471159, "Score"=989.1618691264235}]}  # Ellipses
          n461 = Variant To Data(type=w1070, Variant=w1080) -> (data=w1079:T96)  [unwired: 1 in, 1 out]
          n462 = Unbundle(w1079) -> ("Pixel"=w1078:T103, "Ellipses (Calibrated)"=w1075:T104)
          n463 = for {
            tunnel: w1078 -> [w1108] mode=indexing
            tunnel: w1077 -> [w1110]
            tunnel: w1076 -> [w1109]
            tunnel: w1075 -> [w1106] mode=indexing
            tunnel: w1074 -> [w1107]
            tunnel: [w1104] -> w1073 mode=indexing
            tunnel: [w1099] -> w1072 mode=indexing
            tunnel: w1064 -> [w1098]
            tunnel: w1063 -> [w1097]
            tunnel: [w1092] -> w1066 mode=indexing
            tunnel: w1069 -> [w1088]
            i -> [w1085]
            n464 = Increment(x=w1085) -> (x+1=w1086:i32)
            n465 = Number To Decimal String(number=w1086) -> (decimal integer string=w1084:string)  [unwired: 1 in]
            n466 = Concatenate Strings(w1088, "Ellipses" ("string"), w1084) -> (w1087:string)
            n467 = Unbundle By Name(w1108) -> ("Position.X"=w1112:sgl, "Position.Y"=w1111:sgl)  [unwired: 2 out]
            n468 = Add(x=w1109, y=w1111) -> (x+y=w1081:sgl)
            n469 = Add(x=w1110, y=w1112) -> (x+y=w1091:sgl)
            n470 = Bundle(w1091, w1081) -> (w1082:cluster{sgl, sgl})  [unwired: 1 in]
            n471 = call "IMAQ Convert Pixel to Real World"("Pixel Coordinates"=w1082, "Calibrated Image"=w1107) -> ("error out"=w1083:errorcluster, "Real World Coordinates"=w1103:cluster{"X":sgl, "Y":sgl})  [unwired: 4 in, 4 out]
            n472 = Bundle By Name(cluster=w1108, "Position.X"=w1091, "Position.Y"=w1081) -> (w1095:T105)
            n473 = Bundle By Name(cluster=w1106, "Position"=w1103) -> (w1093:T106)
            n474 = Bundle(w1091, w1081) -> (w1090:cluster{sgl, sgl})  [unwired: 1 in]
            n475 = Unbundle(w1103) -> ("X"=w1101:sgl, "Y"=w1100:sgl)
            n476 = Bundle(cluster=cluster{string, "X":dbl, "Y":dbl} {"", "X"=0.0, "Y"=0.0}, w1087, "X"=w1091, "Y"=w1081) -> (w1104:cluster{string, "X":dbl, "Y":dbl})
            n477 = call "IMAQ Convert Point to ROI"("Point"=w1090) -> ("ROI Descriptor"=w1096:T12)  [unwired: 8 in, 1 out]
            n478 = call <vilib>:"Clear Errors.vi"("error in (no error)"=w1083) -> ()  [unwired: 5 in, 2 out]
            n479 = Bundle(cluster=cluster{string, "X":dbl, "Y":dbl} {"", "X"=0.0, "Y"=0.0}, w1087, "X"=w1101, "Y"=w1100) -> (w1099:cluster{string, "X":dbl, "Y":dbl})
            n480 = call "IMAQ TransformROI"("New Reference"=w1097, "Base Reference"=w1098, "ROI Descriptor"=w1096) -> ("ROI Descriptor out"=w1094:T12)  [unwired: 7 in, 1 out]
            n481 = Bundle("ROI Descriptor out"=w1094, "Circle Descriptor"=w1095, "Circle Descriptor"=w1093) -> (w1092:T107)  [unwired: 1 in]
          }
          n482 = Bundle("Enum_ShapeType"=w1068, "DectectItem"=w1067, w1066) -> (w1065:T108)  [unwired: 1 in]
          n483 = To Variant(anything=w1065) -> (Variant=w1071:variant)
        }
        frame "Lines" {
          w1120 = T109 {"Lines"=[{"Start Point"={"X"=71.38085, "Y"=418.0}, "End Point"={"X"=87.84137, "Y"=435.0}, "Length"=24.758836806279895, "Angle"=314.0763032841935, "Score"=996.0169534496804}], "Lines Calibrated"=[{"Start Point"={"X"=71.38085, "Y"=418.0}, "End Point"={"X"=87.84137, "Y"=435.0}, "Length"=24.758836806279895, "Orientation"=314.0763032841935, "Score"=996.0169534496804}]}  # Lines
          n484 = Variant To Data(type=w1120, Variant=w1132) -> (data=w1131:T109)  [unwired: 1 in, 1 out]
          n485 = Unbundle(w1131) -> ("Lines"=w1130:T110, "Lines Calibrated"=w1127:T111)
          n486 = for {
            tunnel: w1130 -> [w1165] mode=indexing
            tunnel: w1129 -> [w1185]
            tunnel: w1128 -> [w1183]
            tunnel: w1127 -> [w1157] mode=indexing
            tunnel: w1126 -> [w1195]
            tunnel: w1119 -> [w1191]
            tunnel: w1123 -> [w1173]
            tunnel: w1122 -> [w1172]
            tunnel: [w1154] -> w1114 mode=indexing
            shift-right: [w1178] -> w1125
            shift-left: cluster{string, "X":dbl, "Y":dbl}[] [] -> [w1136]
            shift-right: [w1137] -> w1124
            shift-left: cluster{string, "X":dbl, "Y":dbl}[] [] -> [w1135]
            i -> [w1192]
            n487 = Increment(x=w1192) -> (x+1=w1193:i32)
            n488 = Unbundle By Name(w1165) -> ("Start Point.X"=w1197:sgl, "Start Point.Y"=w1196:sgl, "End Point.X"=w1184:sgl, "End Point.Y"=w1182:sgl, "Length"=w1164:dbl, "Angle"=w1163:dbl, "Score"=w1162:dbl)
            n489 = Number To Decimal String(number=w1193) -> (decimal integer string=w1189:string)  [unwired: 1 in]
            n490 = Add(x=w1183, y=w1196) -> (x+y=w1176:sgl)
            n491 = Add(x=w1185, y=w1197) -> (x+y=w1177:sgl)
            n492 = Add(x=w1183, y=w1182) -> (x+y=w1174:sgl)
            n493 = Add(x=w1185, y=w1184) -> (x+y=w1175:sgl)
            n494 = Concatenate Strings(w1191, "Line" ("string"), w1189) -> (w1187:string)
            n495 = Bundle(w1177, w1176) -> (w1166:cluster{sgl, sgl})  [unwired: 1 in]
            n496 = Bundle(w1175, w1174) -> (w1160:cluster{sgl, sgl})  [unwired: 1 in]
            n497 = call "IMAQ Convert Point to ROI"("Point"=w1166) -> ("ROI Descriptor"=w1171:T12)  [unwired: 8 in, 1 out]
            n498 = call "IMAQ Convert Point to ROI"("Point"=w1160) -> ("ROI Descriptor"=w1170:T12)  [unwired: 8 in, 1 out]
            n499 = call "IMAQ TransformROI"("New Reference"=w1172, "Base Reference"=w1173, "ROI Descriptor"=w1170) -> ("ROI Descriptor out"=w1167:T12)  [unwired: 7 in, 1 out]
            n500 = call "IMAQ TransformROI"("New Reference"=w1172, "Base Reference"=w1173, "ROI Descriptor"=w1171) -> ("error out"=w1169:errorcluster, "ROI Descriptor out"=w1168:T12)  [unwired: 7 in]
            n501 = Concatenate Strings(w1187, ".P1" ("string")) -> (w1145:string)
            n502 = call "IMAQ Convert ROI to Point"("error in (no error)"=w1169, "ROI Descriptor"=w1168) -> ("Point"=w1151:T15)  [unwired: 7 in, 1 out]
            n503 = call "IMAQ Convert ROI to Point"("ROI Descriptor"=w1167) -> ("Point"=w1150:T15)  [unwired: 8 in, 1 out]
            n504 = call "IMAQ Convert Pixel to Real World"("Pixel Coordinates"=w1151, "Calibrated Image"=w1195) -> ("error out"=w1134:errorcluster, "Real World Coordinates"=w1159:cluster{"X":sgl, "Y":sgl}, "Calibrated Image (duplicate)"=w1161:T2)  [unwired: 4 in, 3 out]
            n505 = Concatenate Strings(w1187, ".P2" ("string")) -> (w1144:string)
            n506 = Unbundle(w1151) -> ("X"=w1153:sgl, "Y"=w1152:sgl)
            n507 = call "IMAQ Convert Pixel to Real World"("error in (no error)"=w1134, "Pixel Coordinates"=w1150, "Calibrated Image"=w1161) -> ("error out"=w1133:errorcluster, "Real World Coordinates"=w1158:cluster{"X":sgl, "Y":sgl})  [unwired: 3 in, 4 out]
            n508 = Unbundle(w1150) -> ("X"=w1149:sgl, "Y"=w1148:sgl)
            n509 = call <vilib>:"Clear Errors.vi"("error in (no error)"=w1133) -> ()  [unwired: 5 in, 2 out]
            n510 = Bundle(cluster=cluster{string, "X":dbl, "Y":dbl} {"", "X"=0.0, "Y"=0.0}, w1145, "X"=w1153, "Y"=w1152) -> (w1180:cluster{string, "X":dbl, "Y":dbl})
            n511 = Unbundle(w1158) -> ("X"=w1141:sgl, "Y"=w1140:sgl)
            n512 = Bundle(cluster=cluster{string, "X":dbl, "Y":dbl} {"", "X"=0.0, "Y"=0.0}, w1144, "X"=w1149, "Y"=w1148) -> (w1179:cluster{string, "X":dbl, "Y":dbl})
            n513 = Unbundle(w1159) -> ("X"=w1143:sgl, "Y"=w1142:sgl)
            n514 = Bundle By Name(cluster=w1165, "Start Point.X"=w1153, "Start Point.Y"=w1152, "End Point.X"=w1149, "End Point.Y"=w1148, "Length"=w1164, "Angle"=w1163, "Score"=w1162) -> (w1155:T112)
            n515 = Build Array (concatenate)(w1136, w1180, w1179) -> (w1178:cluster{string, "X":dbl, "Y":dbl}[])
            n516 = Bundle By Name(cluster=w1157, "Start Point.X"=w1143, "Start Point.Y"=w1142, "End Point.X"=w1141, "End Point.Y"=w1140) -> (w1156:T113)
            n517 = Bundle("Circle Descriptor"=w1155, "Circle Descriptor"=w1156) -> (w1154:T114)  [unwired: 1 in]
            n518 = Bundle(cluster=cluster{string, "X":dbl, "Y":dbl} {"", "X"=0.0, "Y"=0.0}, w1145, "X"=w1143, "Y"=w1142) -> (w1138:cluster{string, "X":dbl, "Y":dbl})
            n519 = Bundle(cluster=cluster{string, "X":dbl, "Y":dbl} {"", "X"=0.0, "Y"=0.0}, w1144, "X"=w1141, "Y"=w1140) -> (w1139:cluster{string, "X":dbl, "Y":dbl})
            n520 = Build Array (concatenate)(w1135, w1138, w1139) -> (w1137:cluster{string, "X":dbl, "Y":dbl}[])
          }
          n521 = Bundle("Enum_ShapeType"=w1116, "DectectItem"=w1115, w1114) -> (w1113:T115)  [unwired: 1 in]
          n522 = To Variant(anything=w1113) -> (Variant=w1121:variant)
        }
        frame "Rectangles" {
          w1203 = T116 {"Rectangles"=[{"Corners"=[{"X"=1246.2902, "Y"=112.645035}, {"X"=1747.8695, "Y"=51.553356}, {"X"=1809.5117, "Y"=552.8805}, {"X"=1308.092, "Y"=614.1959}, {"X"=1246.2902, "Y"=112.645035}], "Angle"=353.0556571411225, "Width"=505.286090479947, "Height"=505.1026238059605, "Score"=995.1308308658812}], "Rectangles Calibrated"=[{"Corners"=[{"X"=1246.2902, "Y"=112.645035}, {"X"=1747.8695, "Y"=51.553356}, {"X"=1809.5117, "Y"=552.8805}, {"X"=1308.092, "Y"=614.1959}, {"X"=1246.2902, "Y"=112.645035}], "Angle"=353.0556571411225, "Width"=505.286090479947, "Height"=505.1026238059605, "Score"=995.1308308658812}]}  # Rectangles
          n523 = Variant To Data(type=w1203, Variant=w1218) -> (data=w1217:T116)  [unwired: 1 in, 1 out]
          n524 = Unbundle(w1217) -> ("Rectangles"=w1216:T117, "Rectangles Calibrated"=w1213:T117)
          n525 = for {
            tunnel: w1216 -> [w1233] mode=indexing
            tunnel: w1215 -> [w1237]
            tunnel: w1214 -> [w1236]
            tunnel: w1213 -> [w1232] mode=indexing
            tunnel: w1212 -> [w1243]
            tunnel: w1206 -> [w1240]
            tunnel: w1209 -> [w1235]
            tunnel: w1208 -> [w1234]
            tunnel: [w1229] -> w1201 mode=indexing
            shift-right: [w1226] -> w1211
            shift-left: cluster{string, "X":dbl, "Y":dbl}[] [] -> [w1225]
            shift-right: [w1223] -> w1210
            shift-left: cluster{string, "X":dbl, "Y":dbl}[] [] -> [_]
            tunnel: w1199 -> [w1222]
            i -> [w1241]
            n526 = Increment(x=w1241) -> (x+1=w1242:i32)
            n527 = Unbundle By Name(w1233) -> ("Corners"=w1228:cluster{"X":sgl, "Y":sgl}[])
            n528 = Number To Decimal String(number=w1242) -> (decimal integer string=w1238:string)  [unwired: 1 in]
            n529 = for {
              tunnel: w1237 -> [w1283]
              tunnel: w1236 -> [w1282]
              tunnel: w1235 -> [w1279]
              tunnel: w1234 -> [w1278]
              tunnel: [w1273] -> w1220 mode=indexing
              tunnel: w1228 -> [w1272] mode=indexing
              n530 = Unbundle(w1272) -> ("X"=w1271:sgl, "Y"=w1270:sgl)
              n531 = Add(x=w1283, y=w1271) -> (x+y=w1281:sgl)
              n532 = Add(x=w1282, y=w1270) -> (x+y=w1280:sgl)
              n533 = Bundle(w1281, w1280) -> (w1274:cluster{sgl, sgl})  [unwired: 1 in]
              n534 = call "IMAQ Convert Point to ROI"("Point"=w1274) -> ("ROI Descriptor"=w1277:T12)  [unwired: 8 in, 1 out]
              n535 = call "IMAQ TransformROI"("New Reference"=w1278, "Base Reference"=w1279, "ROI Descriptor"=w1277) -> ("error out"=w1276:errorcluster, "ROI Descriptor out"=w1275:T12)  [unwired: 7 in]
              n536 = call "IMAQ Convert ROI to Point"("error in (no error)"=w1276, "ROI Descriptor"=w1275) -> ("Point"=w1273:T15)  [unwired: 7 in, 1 out]
            }
            n537 = Concatenate Strings(w1240, "Rectangles" ("string"), w1238) -> (w1224:string)
            n538 = for {
              tunnel: w1243 -> [w1269]
              tunnel: [w1268] -> w1221 mode=indexing
              tunnel: w1220 -> [w1267] mode=indexing
              n539 = call "IMAQ Convert Pixel to Real World"("Pixel Coordinates"=w1267, "Calibrated Image"=w1269) -> ("error out"=w1266:errorcluster, "Real World Coordinates"=w1268:cluster{"X":sgl, "Y":sgl})  [unwired: 4 in, 4 out]
              n540 = call <vilib>:"Clear Errors.vi"("error in (no error)"=w1266) -> ()  [unwired: 5 in, 2 out]
            }
            n541 = Select(t=w1221, s=w1222, f=w1220) -> (s? t:f=w1219:T15[])
            n542 = for {
              tunnel: w1224 -> [w1248]
              tunnel: w1219 -> [w1247] mode=indexing
              tunnel: [w1244] -> w1223 mode=indexing
              i -> [w1253]
              n543 = Increment(x=w1253) -> (x+1=w1252:i32)
              n544 = Unbundle(w1247) -> ("X"=w1246:sgl, "Y"=w1245:sgl)
              n545 = Number To Decimal String(number=w1252) -> (decimal integer string=w1250:string)  [unwired: 1 in]
              n546 = Concatenate Strings(w1248, ".P" ("string"), w1250) -> (w1249:string)
              n547 = Bundle(cluster=cluster{string, "X":dbl, "Y":dbl} {"", "X"=0.0, "Y"=0.0}, w1249, "X"=w1246, "Y"=w1245) -> (w1244:cluster{string, "X":dbl, "Y":dbl})
            }
            n548 = Bundle By Name(cluster=w1233, "Corners"=w1220) -> (w1230:T118)
            n549 = for {
              tunnel: w1224 -> [w1259]
              tunnel: w1220 -> [w1258] mode=indexing
              tunnel: [w1255] -> w1227 mode=indexing
              i -> [w1264]
              n550 = Increment(x=w1264) -> (x+1=w1263:i32)
              n551 = Unbundle(w1258) -> ("X"=w1257:sgl, "Y"=w1256:sgl)
              n552 = Number To Decimal String(number=w1263) -> (decimal integer string=w1261:string)  [unwired: 1 in]
              n553 = Concatenate Strings(w1259, ".P" ("string"), w1261) -> (w1260:string)
              n554 = Bundle(cluster=cluster{string, "X":dbl, "Y":dbl} {"", "X"=0.0, "Y"=0.0}, w1260, "X"=w1257, "Y"=w1256) -> (w1255:cluster{string, "X":dbl, "Y":dbl})
            }
            n555 = Bundle By Name(cluster=w1232, "Corners"=w1221) -> (w1231:T118)
            n556 = Bundle("Rectangle Descriptor"=w1230, "Rectangle Descriptor"=w1231) -> (w1229:T119)  [unwired: 1 in]
            n557 = Build Array (concatenate)(w1225, w1227) -> (w1226:cluster{string, "X":dbl, "Y":dbl}[])
          }
          n558 = Bundle("Enum_ShapeType"=w1202, "DectectItem"=w1198, w1201) -> (w1200:T120)  [unwired: 1 in]
          n559 = To Variant(anything=w1200) -> (Variant=w1207:variant)
        }
      }
    }
    frame 12 {
      n560 = Concatenate Strings(w1293, "_" ("string"), w1291) -> (w1290:string)
      n561 = Variant To Data(type=T28 {"OCRSelectedLanaguage"=[]} ("OCR_Setting Parameter"), Variant=w1284) -> (data=w1294:T28)  [unwired: 1 in, 1 out]
      n562 = Unbundle By Name(w1294) -> ("OCRSelectedLanaguage"=w1289:string[])
      n563 = Empty Array?(array=w1289) -> (empty?=w1288:bool)
      n564 = case shown="False" w1288 {
        tunnel: w1286 -> [w1309 _]
        tunnel: w1290 -> [w1297 _]
        tunnel: w1289 -> [w1301 _]
        tunnel: [w1296 _] -> w1287
        frame False {
          w1298 = path "C:/Smasoft/System"
          n565 = call "OCR_Main_Function.vi"("Item Names"=w1301, "String"=w1297, "Refnum in"=w1309) -> ("error out"=w1300:errorcluster)  [unwired: 8 in]
          n566 = Concatenate Strings(w1297, ".txt" ("string")) -> (w1307:string)
          n567 = Build Path(base path=w1298, name or relative path=w1307) -> (appended path=w1306:path)
          n568 = Open/Create/Replace File(file path (use dialog)=w1306, error in=w1300) -> (refnum out=w1305:refnum<file>, error out=w1304:errorcluster)  [unwired: 4 in, 1 out]
          n569 = Read from Text File(file (use dialog)=w1305, error in=w1304) -> (refnum out=w1303:refnum<file>, text=w1299:string, error out=w1302:errorcluster)  [unwired: 2 in, 1 out]
          n570 = disable-structure shown="Enabled" {
            disable-tunnel: w1303 -> [w1324 _]
            disable-tunnel: w1302 -> [w1323 _]
            disable-tunnel: w1298 -> [w1314 _]
            disable-tunnel: w1297 -> [w1313 _]
            frame Disabled {
              n571 = Close File(refnum=w1324, error in=w1323) -> (error out=w1312:errorcluster)  [unwired: 1 out]
              n572 = Concatenate Strings(w1313, ".tiff" ("string")) -> (w1321:string)
              n573 = Concatenate Strings(w1313, ".txt" ("string")) -> (w1319:string)
              n574 = Build Path(base path=w1314, name or relative path=w1319) -> (appended path=w1317:path)
              n575 = Build Path(base path=w1314, name or relative path=w1321) -> (appended path=w1318:path)
              n576 = call <vilib>:"Check if File or Folder Exists.vi"("error in (no error)"=w1312, "path"=w1318) -> ("file or folder exists?"=w1316:bool, "dup path"=w1315:path)  [unwired: 7 in, 1 out]
              n577 = call <vilib>:"Check if File or Folder Exists.vi"("error in (no error)"=w1312, "path"=w1317) -> ("file or folder exists?"=w1311:bool, "dup path"=w1310:path)  [unwired: 7 in, 1 out]
              n578 = case shown="True" w1311 {
                tunnel: w1310 -> [_ w1325]
                frame False {
                }
                frame True {
                  n579 = Delete(path (use dialog)=w1325) -> ()  [unwired: 4 in, 3 out]
                }
              }
              n580 = case shown="True" w1316 {
                tunnel: w1315 -> [_ w1326]
                frame False {
                }
                frame True {
                  n581 = Delete(path (use dialog)=w1326) -> ()  [unwired: 4 in, 3 out]
                }
              }
            }
            frame Enabled {
            }
          }
          n582 = call <vilib>:"Trim Whitespace.vi"("string"=w1299) -> ("trimmed string"=w1296:string)  [unwired: 1 in]
        }
        frame True {
        }
      }
      n583 = To Variant(anything=w1287) -> (Variant=w1285:variant)
    }
    frame 13 {
      w1345 = T121 {"ROI"={"Global Rectangle"=[], "Contours"=[]}, "Search Direction"=enum."Rect Left To Right", "Curve Extraction"={"Extraction Mode"=0, "Edge Threshold"=75, "Edge Filter Size"=1, "Min Length"=25, "Search Step Size"=15, "Max Endpoint Gap"=10, "Subpixel"=TRUE}, "Contour Selection"=enum."Closest To Search Start", "Curve Connection"=[]}  # ContourParameter
      n584 = Unbundle By Name(w1336) -> ("Reference System"=w1334:T36, "Measurement System"=w1335:T36)
      n585 = Variant To Data(type=w1345, Variant=w1344) -> (data=w1343:T121)  [unwired: 1 in, 1 out]
      n586 = call "Contour.vi"("ContourParameter"=w1343, "Image In"=w1342) -> ("ContourResult"=w1332:T124, "Image Out"=w1328:T2)  [unwired: 7 in, 1 out]
      n587 = Unbundle By Name(w1332) -> ("Points (pixel)"=w1339:cluster{"X":dbl, "Y":dbl}[])  [unwired: 1 out]
      n588 = Bundle(w1341, w1340) -> (w1338:cluster{i32, i32})  [unwired: 1 in]
      n589 = Add(x=w1338, y=w1339) -> (x+y=w1337:cluster{dbl, dbl}[])
      n590 = for {
        tunnel: w1337 -> [w1359] mode=indexing
        tunnel: w1335 -> [w1353]
        tunnel: w1334 -> [w1354]
        tunnel: [w1352] -> w1330 mode=indexing
        tunnel: [w1351] -> _
        n591 = call "IMAQ Convert Point to ROI"("Point"=w1359) -> ("error out"=w1355:errorcluster, "ROI Descriptor"=w1356:T12)  [unwired: 8 in]
        n592 = call "IMAQ TransformROI"("error in (no error)"=w1355, "New Reference"=w1353, "Base Reference"=w1354, "ROI Descriptor"=w1356) -> ("error out"=w1358:errorcluster, "ROI Descriptor out"=w1357:T12)  [unwired: 6 in]
        n593 = call "IMAQ Convert ROI to Point"("error in (no error)"=w1358, "ROI Descriptor"=w1357) -> ("error out"=w1351:errorcluster, "Point"=w1352:T15)  [unwired: 7 in]
      }
      n594 = case shown="True" w1333 {
        tunnel: w1328 -> [_ w1350]
        tunnel: w1330 -> [_ w1349]
        tunnel: [cluster{"X":sgl, "Y":sgl}[] [] ("Array of Real World Coordinates") w1347] -> w1331
        frame False {
        }
        frame True {
          n595 = call "IMAQ Convert Pixel to Real World"("Array of Pixel Coordinates"=w1349, "Calibrated Image"=w1350) -> ("error out"=w1348:errorcluster, "Array of Real World Coordinates"=w1347:cluster{"X":sgl, "Y":sgl}[])  [unwired: 4 in, 4 out]
          n596 = call <vilib>:"Clear Errors.vi"("error in (no error)"=w1348) -> ()  [unwired: 5 in, 2 out]
        }
      }
      n597 = Bundle By Name(cluster=w1332, "Points (pixel)"=w1330, "Points (real)"=w1331) -> (w1329:T124)
      n598 = To Variant(anything=w1329) -> (Variant=w1327:variant)
    }
    frame 14 {
      n599 = Unbundle By Name(w1390) -> ("Reference System"=w1388:T36, "Measurement System"=w1389:T36)
      n600 = Variant To Data(type=T30 {"Color Sensitivity"=0, "Learn Saturation Threshold"=80, "Minimum Match Score"=800.0, "Match Saturation Threshold"=80, "ROI Descriptor"={"Global Rectangle"=[], "Contours"=[]}, "TemplatePath"="", "ColorSpectrum"=[]} ("ColorMatchParameter"), Variant=w1392) -> (data=w1365:T30)  [unwired: 1 in, 1 out]
      n601 = Unbundle By Name(w1365) -> ("ROI Descriptor"=w1363:T12, "ROI Descriptor.Global Rectangle"=w1376:i32[], "ROI Descriptor.Contours"=w1378:T125)
      n602 = call "ColorMatch_MainFunction.vi"("ColorMatchParameter"=w1365, "Vision_Image In"=w1391) -> ("Match Score"=w1385:i32[], "Match Flag"=w1386:bool[])  [unwired: 7 in, 1 out]
      n603 = Bundle(w1373, w1370) -> (w1377:cluster{i32, i32})  [unwired: 1 in]
      n604 = Index Array(array=w1376) -> (element #1=w1375:i32, element #2=w1372:i32, element #3=w1374:i32, element #4=w1371:i32)  [unwired: 4 in]
      n605 = for {
        tunnel: w1378 -> [w1396] mode=indexing
        tunnel: w1377 -> [w1399]
        tunnel: [w1394] -> w1361 mode=indexing
        n606 = Unbundle By Name(w1396) -> ("Coordinates"=w1404:i32[])
        n607 = Array Size(array=w1404) -> (size(s)=w1397:i32)
        n608 = Divide(x=w1397, y=2) -> (x/y=w1393:dbl)
        n609 = Round Toward +Infinity(x=w1393) -> (ceil(x): smallest int >= x=w1401:dbl)
        n610 = Reshape Array(w1404, w1401, 2 ("dimension size")) -> (w1400:i32[][])
        n611 = for {
          N: w1401 -> [_]
          tunnel: w1400 -> [w1411] mode=indexing
          tunnel: w1399 -> [w1408]
          tunnel: [w1405] -> w1398 mode=indexing
          n612 = Index Array(array=w1411) -> (element #1=w1410:i32, element #2=w1409:i32)  [unwired: 2 in]
          n613 = Bundle(w1410, w1409) -> (w1407:cluster{i32, i32})  [unwired: 1 in]
          n614 = Add(x=w1408, y=w1407) -> (x+y=w1406:cluster{i32, i32})
          n615 = Cluster To Array(cluster=w1406) -> (array=w1405:i32[])
        }
        n616 = Reshape Array(w1398, w1397) -> (w1395:i32[])
        n617 = Bundle By Name(cluster=w1396, "Coordinates"=w1395) -> (w1394:T126)
      }
      n618 = Add(x=w1375, y=w1373) -> (x+y=w1369:i32)
      n619 = Add(x=w1374, y=w1373) -> (x+y=w1368:i32)
      n620 = Add(x=w1372, y=w1370) -> (x+y=w1367:i32)
      n621 = Add(x=w1371, y=w1370) -> (x+y=w1366:i32)
      n622 = Build Array(w1369, w1368, w1367, w1366) -> (w1362:i32[])
      n623 = Bundle By Name(cluster=w1363, "Global Rectangle"=w1362, "Contours"=w1361) -> (w1364:T12)
      n624 = case shown="True" w1381 {
        tunnel: [cluster{"X":sgl, "Y":sgl}[] [] ("Array of Real World Coordinates") w1416] -> _
        tunnel: w1380 -> [w1412 w1415]
        tunnel: [w1412 w1414] -> w1379
        frame False {
        }
        frame True {
          n625 = call "IMAQ Convert Pixel to Real World"("Calibrated Image"=w1415) -> ("error out"=w1417:errorcluster, "Array of Real World Coordinates"=w1416:cluster{"X":sgl, "Y":sgl}[], "Calibrated Image (duplicate)"=w1414:T2)  [unwired: 5 in, 3 out]
          n626 = call <vilib>:"Clear Errors.vi"("error in (no error)"=w1417) -> ()  [unwired: 5 in, 2 out]
        }
      }
      n627 = call "IMAQ TransformROI"("New Reference"=w1389, "Base Reference"=w1388, "ROI Descriptor"=w1364) -> ("ROI Descriptor out"=w1360:T12)  [unwired: 7 in, 1 out]
      n628 = Bundle(cluster=T29 {"Match Flag"=[], "Match Score"=[], "ROI Descriptor"={"Global Rectangle"=[], "Contours"=[]}} ("output cluster"), "Match Flag"=w1386, "Match Score"=w1385, "ROI Descriptor"=w1360) -> (w1383:T29)
      n629 = To Variant(anything=w1383) -> (Variant=w1382:variant)
    }
  }
  "Image Out" <- w23
  "Result" <- w22
  "Analysis_Point_Result Out" <- w16
  "Analysis_Point_Result Out Overlay" <- w3
  n630 = case shown="No Error" w9 {
    selector: w9 -> [w1418 w1419]
    tunnel: [w1418 w1419] -> w8
    frame No Error {
    }
    frame Error {
    }
  }
  "error out" <- w8
